vi "BRig_RT_panel_Laser2_v1,11.vi"(7 "input_setValues":bool, 9 "input_dataExp":u16[](array[numeric]), 11 "input_dataLC":u16[](array[numeric])) -> (1 "output_dataExp":u16[](array[numeric]), 3 "output_dataLC":u16[](array[numeric]))   [LabVIEW 2014]
panel:
  in  "LC_Sel_nRew2":u16
  in  "LC_Sel_nRew1":u16
  in  "LC_Cue2_nRew2":u16
  in  "LC_Cue2_nRew1":u16
  in  "LC_Cue_nRew2":u16
  in  "LC_Cue_nRew1":u16
  in  "LC_ENL2_nRew2":u16
  in  "LC_ENL2_nRew1":u16
  in  "LC_ENL_nRew2":u16
  in  "LC_ENL_nRew1":u16
  in  "LC_Cue2_PostR_Count":u16
  in  "LC_Cue2_PostR_delayOpt":bool
  in  "LC_Cue2_PostR_Probability":u16
  in  "LC_Cue2_PostR_Block":u16(slide) max=2 step=1 scale=0.0..2.0
  in  "LC_Cue2_PostR_OnOff":bool
  in  "LC_Cue2_PostR_Tdelay":u16
  in  "LC_ENL2_PostR_delayOpt":bool
  in  "LC_ENL2_PostR_Count":u16
  in  "LC_ENL2_PostR_Probability":u16 max=100 step=1
  in  "LC_ENL2_PostR_Block":u16(slide) max=2 step=1 scale=0.0..2.0
  in  "LC_ENL2_PostR_OnOff":bool
  in  "LC_ENL2_PostR_Tdelay":u16
  in  "LC_Cue2_PreR_Count":u16
  in  "LC_Cue2_First_Count":u16
  in  "LC_Cue2_PreR_delayOpt":bool
  in  "LC_ENL2_PreR_delayOpt":bool
  in  "LC_ENL2_PreR_Count":u16
  in  "LC_ENL2_First_Count":u16
  in  "LC_Cue2_First_delayOpt":bool
  in  "LC_ENL2_First_delayOpt":bool
  in  "LC_Cue2_PreR_Probability":u16
  in  "LC_Cue2_PreR_Block":u16(slide) max=2 step=1 scale=0.0..2.0
  in  "LC_Cue2_PreR_OnOff":bool
  in  "LC_Cue2_First_Probability":u16
  in  "LC_Cue2_First_Block":u16(slide) max=2 step=1 scale=0.0..2.0
  in  "LC_Cue2_First_OnOff":bool
  in  "LC_ENL2_PreR_Probability":u16 max=100 step=1
  in  "LC_ENL2_PreR_Block":u16(slide) max=2 step=1 scale=0.0..2.0
  in  "LC_ENL2_PreR_OnOff":bool
  in  "LC_ENL2_First_Probability":u16 max=100 step=1
  in  "LC_ENL2_First_Block":u16(slide) max=2 step=1 scale=0.0..2.0
  in  "LC_Cue2_PreR_Tdelay":u16
  in  "LC_ENL2_PreR_Tdelay":u16
  in  "LC_Cue2_First_Tdelay":u16
  in  "LC_ENL2_First_Tdelay":u16
  in  "LC_ENL2_First_OnOff":bool
  out "LaserPulseTrain":cluster{u16[], u16[]}(graph)
  in  "LED_baseline":bool
  in  "Laser_power_step":dbl
  in  "Laser_power_max":dbl
  in  "Laser_power_min":dbl
  in  "Laser_Tshutter":u16=2
  in  "Laser_Freq":u16=10
  in  "Laser_Tpeak":u16=2
  in  "Laser_T":u16
  in  "LC_Sel_PostR_Count":u16
  in  "LC_Sel_PostR_Probability":u16
  in  "LC_Sel_PostR_Block":u16(slide) max=2 step=1 scale=0.0..2.0
  in  "LC_Sel_PostR_OnOff":bool
  in  "LC_Sel_PostR_Tdelay":u16
  in  "LC_Cue_PostR_Count":u16
  in  "LC_Cue_PostR_delayOpt":bool
  in  "LC_Cue_PostR_Probability":u16
  in  "LC_Cue_PostR_Block":u16(slide) max=2 step=1 scale=0.0..2.0
  in  "LC_Cue_PostR_OnOff":bool
  in  "LC_Cue_PostR_Tdelay":u16
  in  "LC_ENL_PostR_delayOpt":bool
  in  "LC_ENL_PostR_Count":u16
  in  "LC_ENL_PostR_Probability":u16 max=100 step=1
  in  "LC_ENL_PostR_Block":u16(slide) max=2 step=1 scale=0.0..2.0
  in  "LC_ENL_PostR_OnOff":bool
  in  "LC_ENL_PostR_Tdelay":u16
  in  "LC_Sel_PreR_Count":u16
  in  "LC_Sel_First_Count":u16
  in  "LC_Sel_PreR_Probability":u16
  in  "LC_Sel_PreR_Block":u16(slide) max=2 step=1 scale=0.0..2.0
  in  "LC_Sel_PreR_OnOff":bool
  in  "LC_Sel_First_Probability":u16
  in  "LC_Sel_First_Block":u16(slide) max=2 step=1 scale=0.0..2.0
  in  "LC_Sel_First_OnOff":bool
  in  "LC_Sel_PreR_Tdelay":u16
  in  "LC_Sel_First_Tdelay":u16
  in  "LC_Cue_PreR_Count":u16
  in  "LC_Cue_First_Count":u16
  in  "LC_Cue_PreR_delayOpt":bool
  in  "LC_ENL_PreR_delayOpt":bool
  in  "LC_ENL_PreR_Count":u16
  in  "LC_ENL_First_Count":u16
  in  "LC_Cue_First_delayOpt":bool
  in  "LC_ENL_First_delayOpt":bool
  in  "LC_Wrong_Probability":u16
  in  "LC_Wrong_Trial":u16(slide) max=2 step=1 scale=0.0..2.0
  in  "LC_Wrong_Block":u16(slide) max=2 step=1 scale=0.0..2.0
  in  "LC_Wrong_OnOff":bool
  in  "LC_Reward_Probability":u16
  in  "LC_Reward_Trial":u16(slide) max=2 step=1 scale=0.0..2.0
  in  "LC_Reward_Block":u16(slide) max=2 step=1 scale=0.0..2.0
  in  "LC_Reward_OnOff":bool
  in  "LC_Cue_PreR_Probability":u16
  in  "LC_Cue_PreR_Block":u16(slide) max=2 step=1 scale=0.0..2.0
  in  "LC_Cue_PreR_OnOff":bool
  in  "LC_Cue_First_Probability":u16
  in  "LC_Cue_First_Block":u16(slide) max=2 step=1 scale=0.0..2.0
  in  "LC_Cue_First_OnOff":bool
  in  "LC_ENL_PreR_Probability":u16 max=100 step=1
  in  "LC_ENL_PreR_Block":u16(slide) max=2 step=1 scale=0.0..2.0
  in  "LC_ENL_PreR_OnOff":bool
  in  "LC_ENL_First_Probability":u16 max=100 step=1
  in  "LC_ENL_First_Block":u16(slide) max=2 step=1 scale=0.0..2.0
  in  "LC_Wrong_Tdelay":u16
  in  "LC_Cue_PreR_Tdelay":u16
  in  "LC_ENL_PreR_Tdelay":u16
  in  "LC_Reward_Tdelay":u16
  in  "LC_Cue_First_Tdelay":u16
  in  "LC_ENL_First_Tdelay":u16
  in  "LC_ENL_First_OnOff":bool
  # "Laser2 Control\n                               On/Off      Block        Probability [%]   Delay [ms]                              Count"
  # "On/Off      Block        Probability [%]   Delay [ms]                              Count"
  # "Enforced\nNonLick"
  # "Enforced\nNonLick\n     2"
  # "from end"
  # "from end"
  # "First\nTrial"
  # "First\nTrial"
  # "from start"
  # "from start"
  # "from end"
  # "from end"
  # "PreReward\nTrials"
  # "PreReward\nTrials"
  # "from start"
  # "from start"
  # "from end"
  # "from end"
  # "PostReward\nTrials"
  # "PostReward\nTrials"
  # "from start"
  # "from start"
  # "PostReward Option - Trigger after [X1] or [X2] reward\n                                        (0 = ignore this option)"
  # "PostReward Option - Trigger after [X1] or [X2] reward\n                                        (0 = ignore this option)"
  # "Cue"
  # "Cue\n  2"
  # "from end"
  # "from end"
  # "First\nTrial"
  # "First\nTrial"
  # "from start"
  # "from start"
  # "from end"
  # "from end"
  # "PreReward\nTrials"
  # "PreReward\nTrials"
  # "from start"
  # "from start"
  # "from end"
  # "from end"
  # "PostReward\nTrials"
  # "PostReward\nTrials"
  # "from start"
  # "from start"
  # "PostReward Option - Trigger after [X1] or [X2] reward\n                                        (0 = ignore this option)"
  # "PostReward Option - Trigger after [X1] or [X2] reward\n                                        (0 = ignore this option)"
  # "Selection"
  # "from start"
  # "First\nTrial"
  # "from start"
  # "PreReward\nTrials"
  # "from start"
  # "PostReward\nTrials"
  # "PostReward Option - Trigger after [X1] or [X2] reward\n                                        (0 = ignore this option)"
  # "Laser2 Parameters"
  # "Laser2 Response\n           On/Off      Block           Trial     Probability %  Delay [ms]"
  # "Frequency\n[Hz]"
  # "Selection\nReward"
  # "Timing [ms]\n Duration     Peak Width   Shutter"
  # "Selection\nWrong"
  # "Laser Power [V]\nMin          Max              Step"
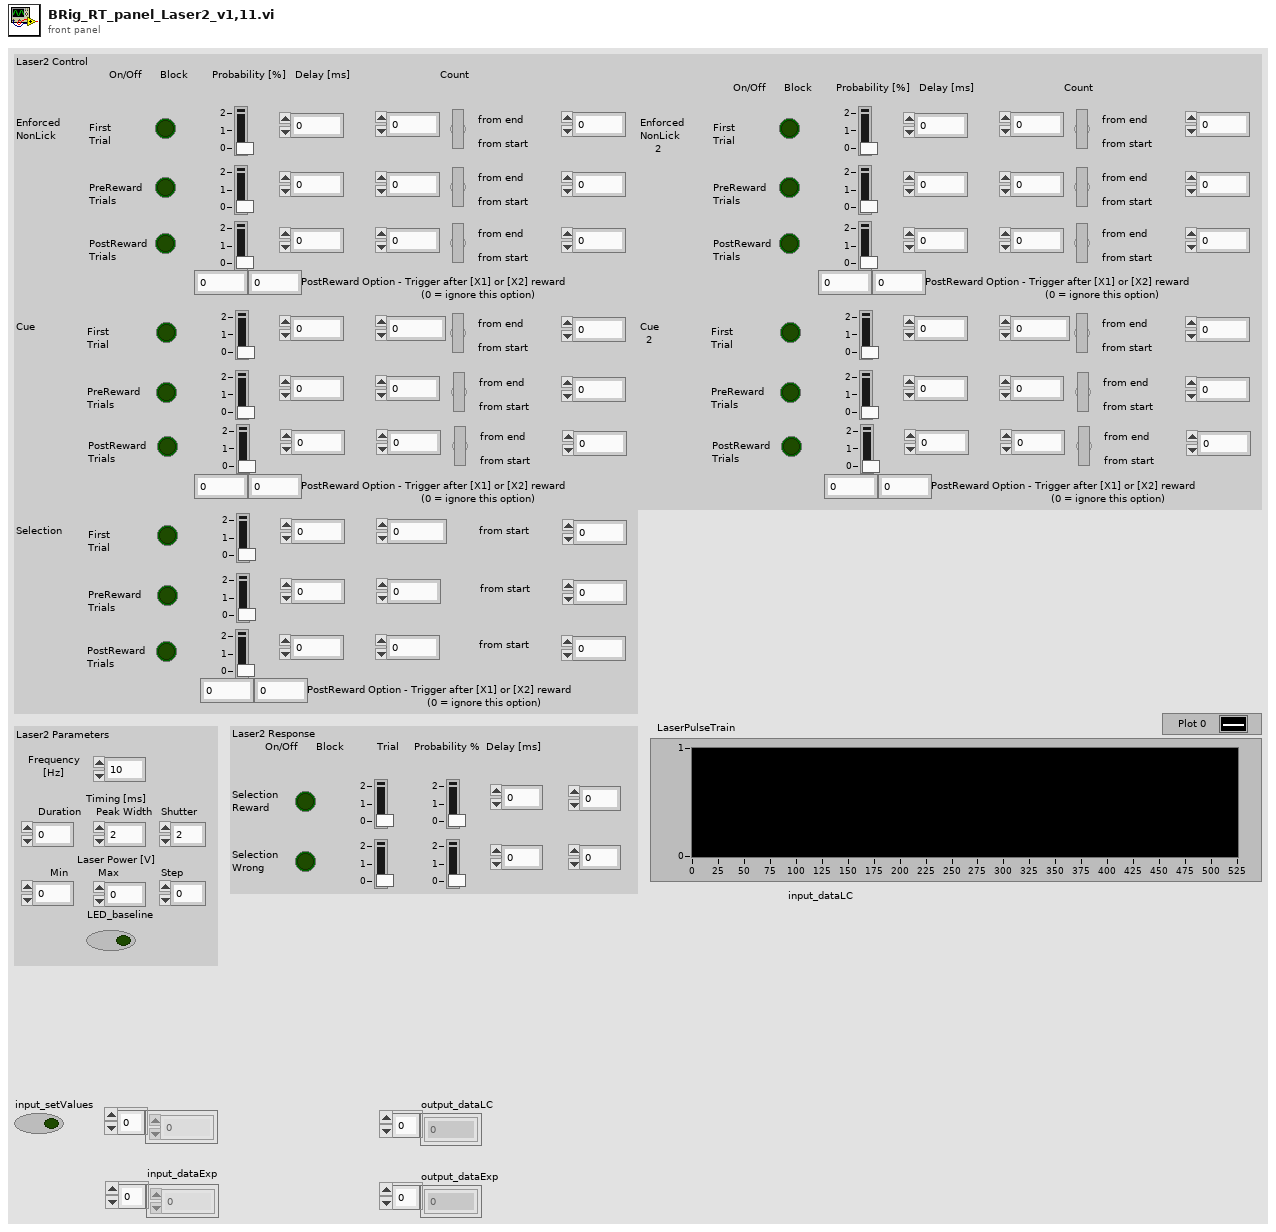
[diagram p1: front panel]
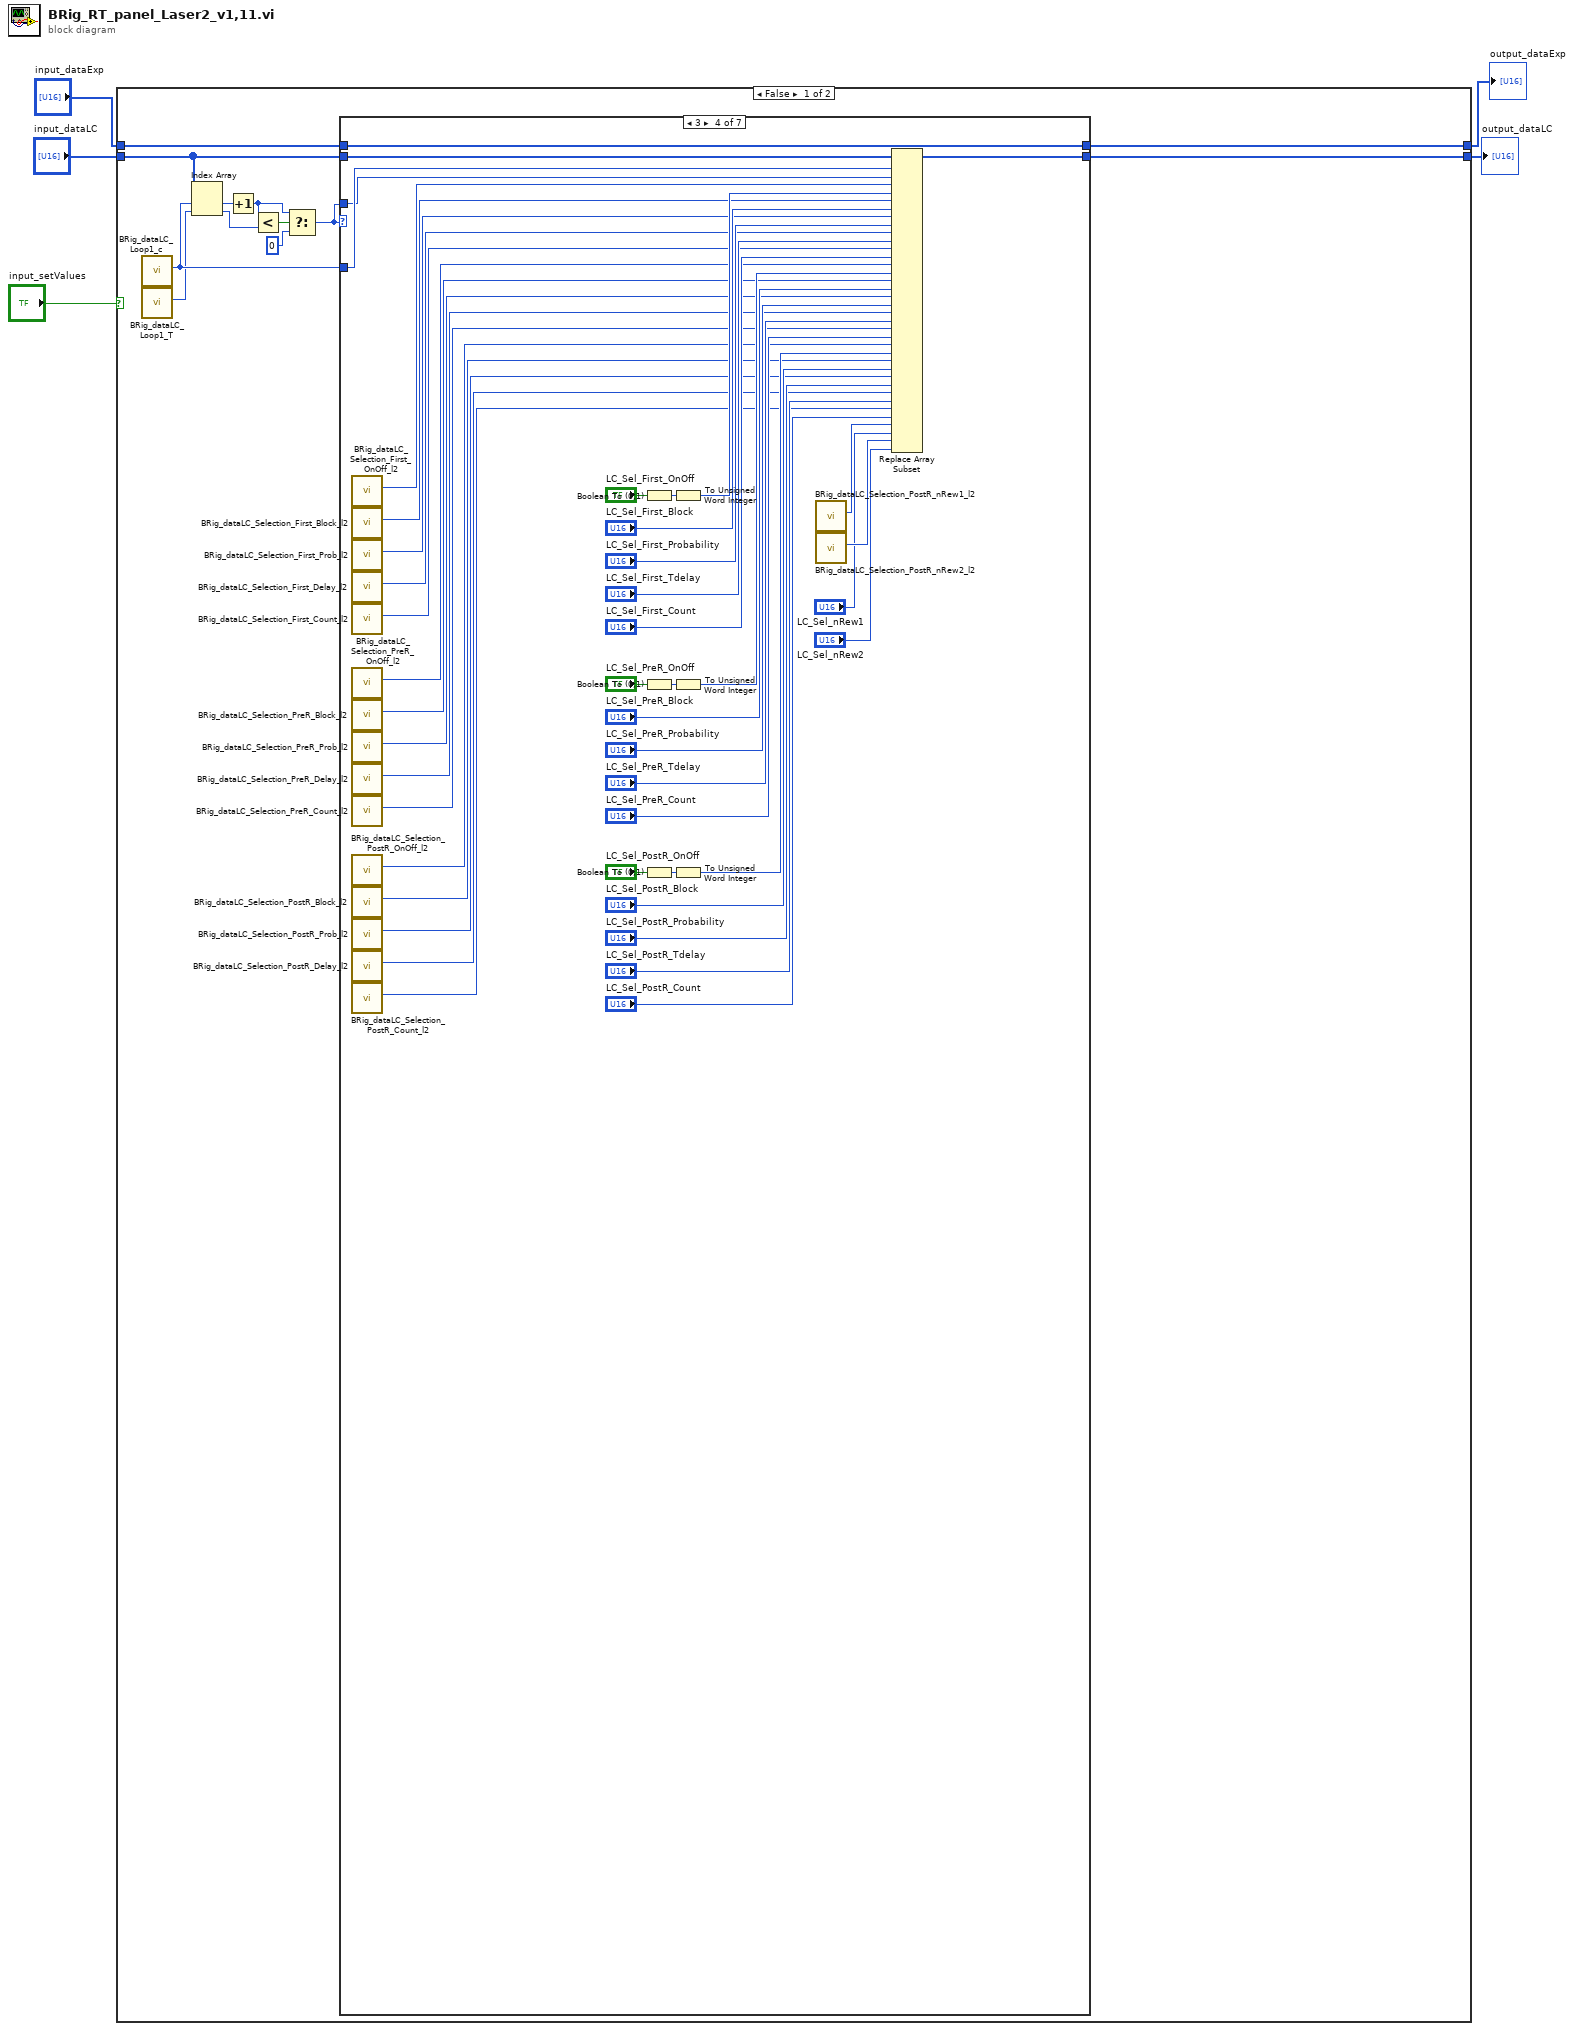
[diagram p0: block diagram]
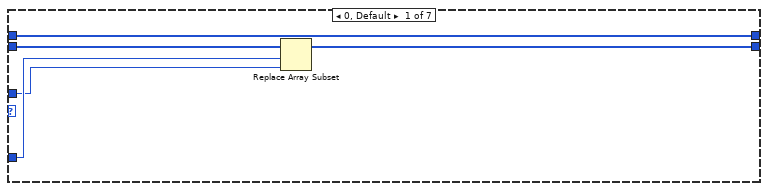
[diagram p2: hidden frame]
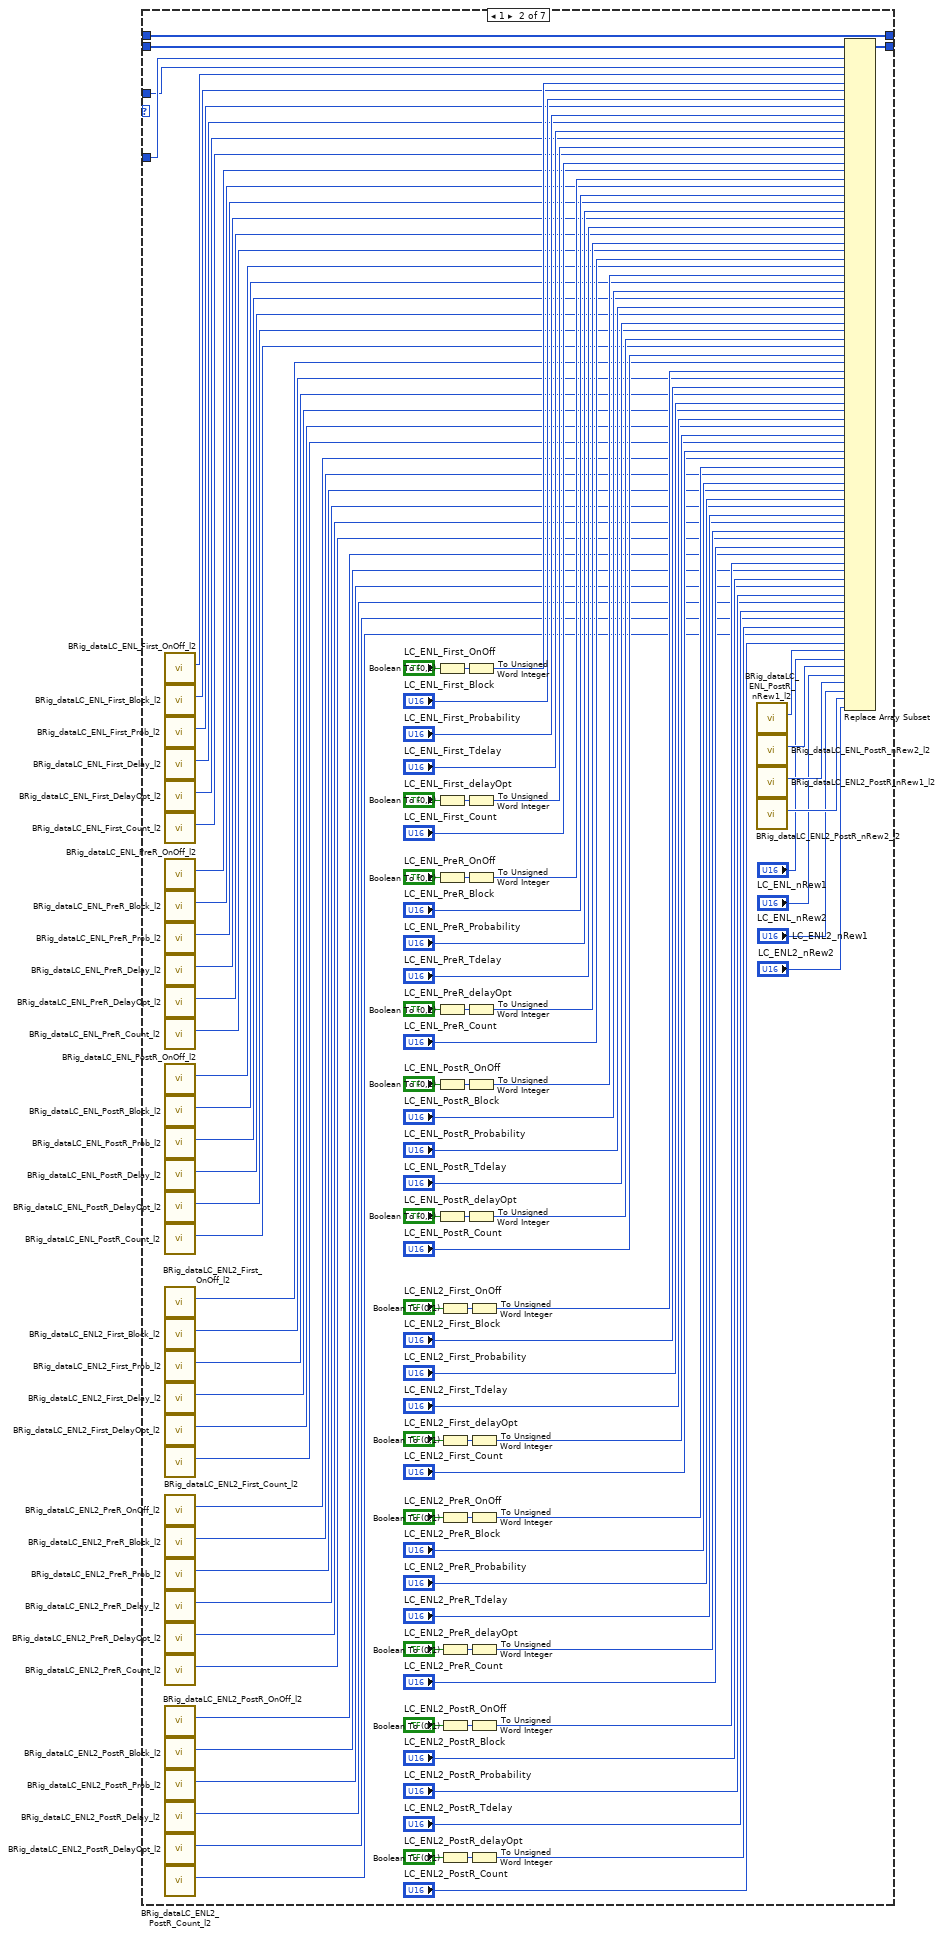
[diagram p3: hidden frame]
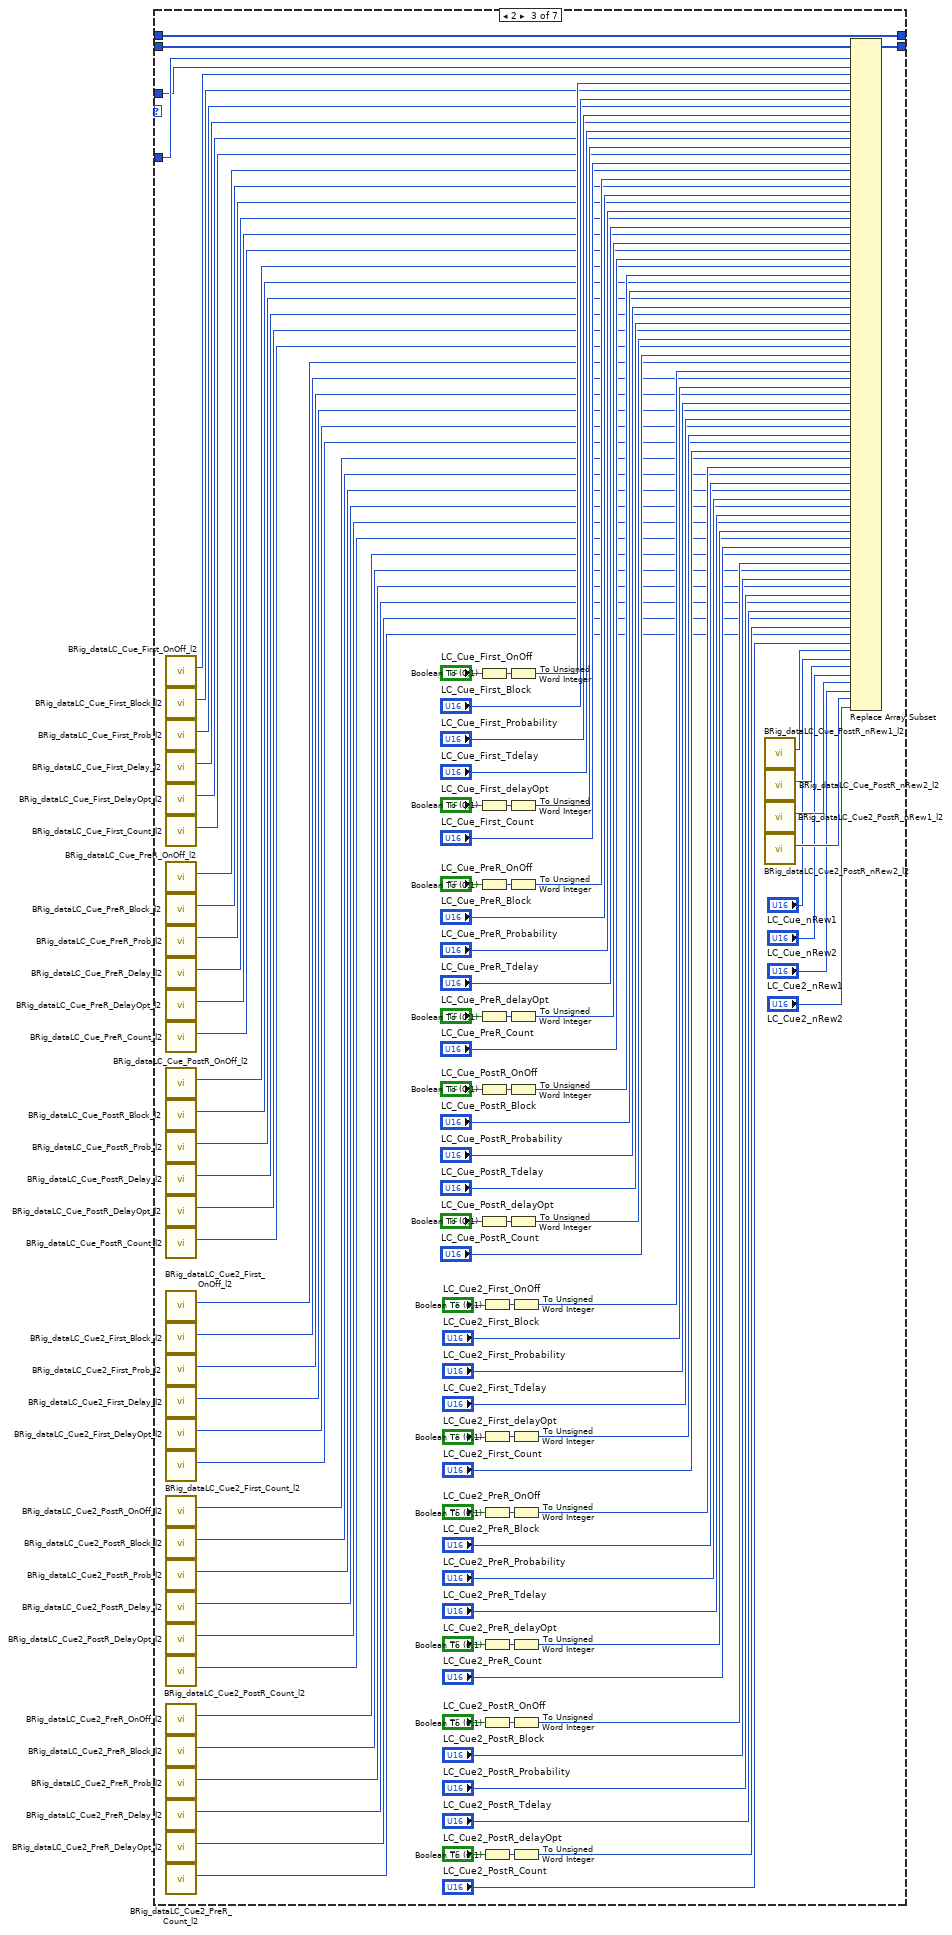
[diagram p4: hidden frame]
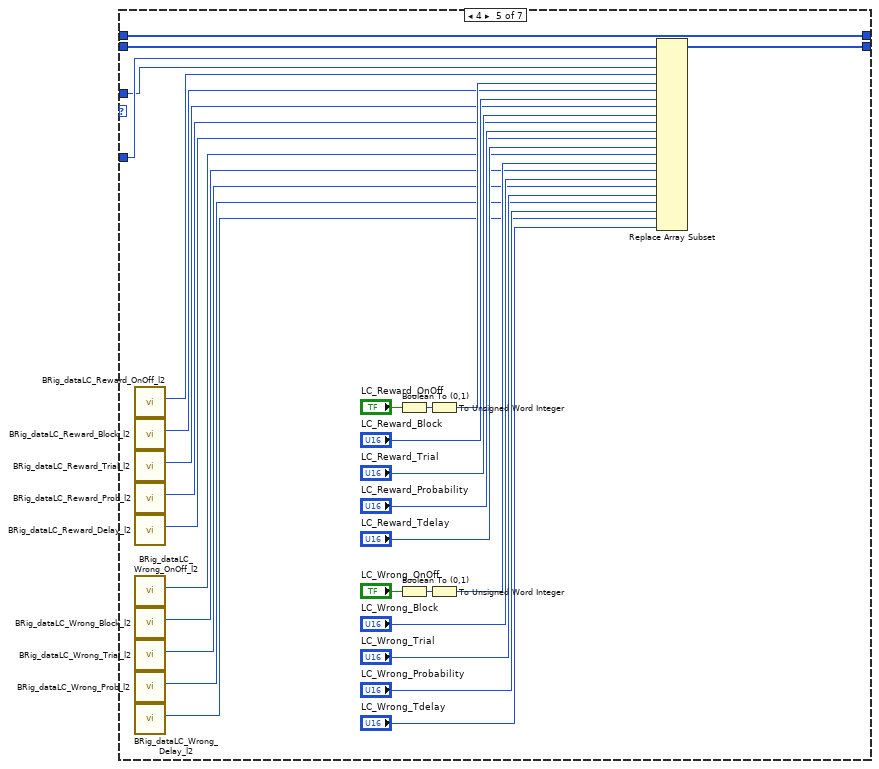
[diagram p5: hidden frame]
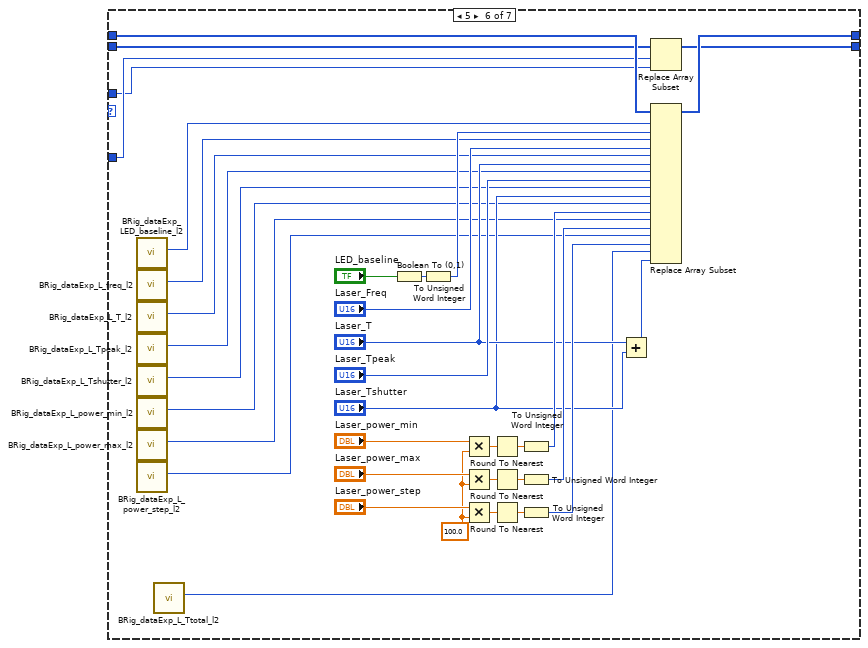
[diagram p6: hidden frame]
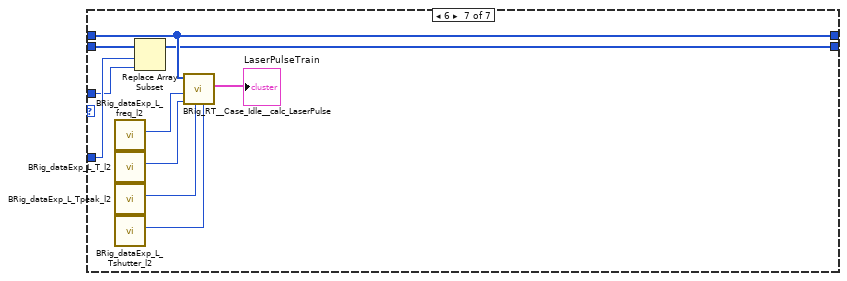
[diagram p7: hidden frame]
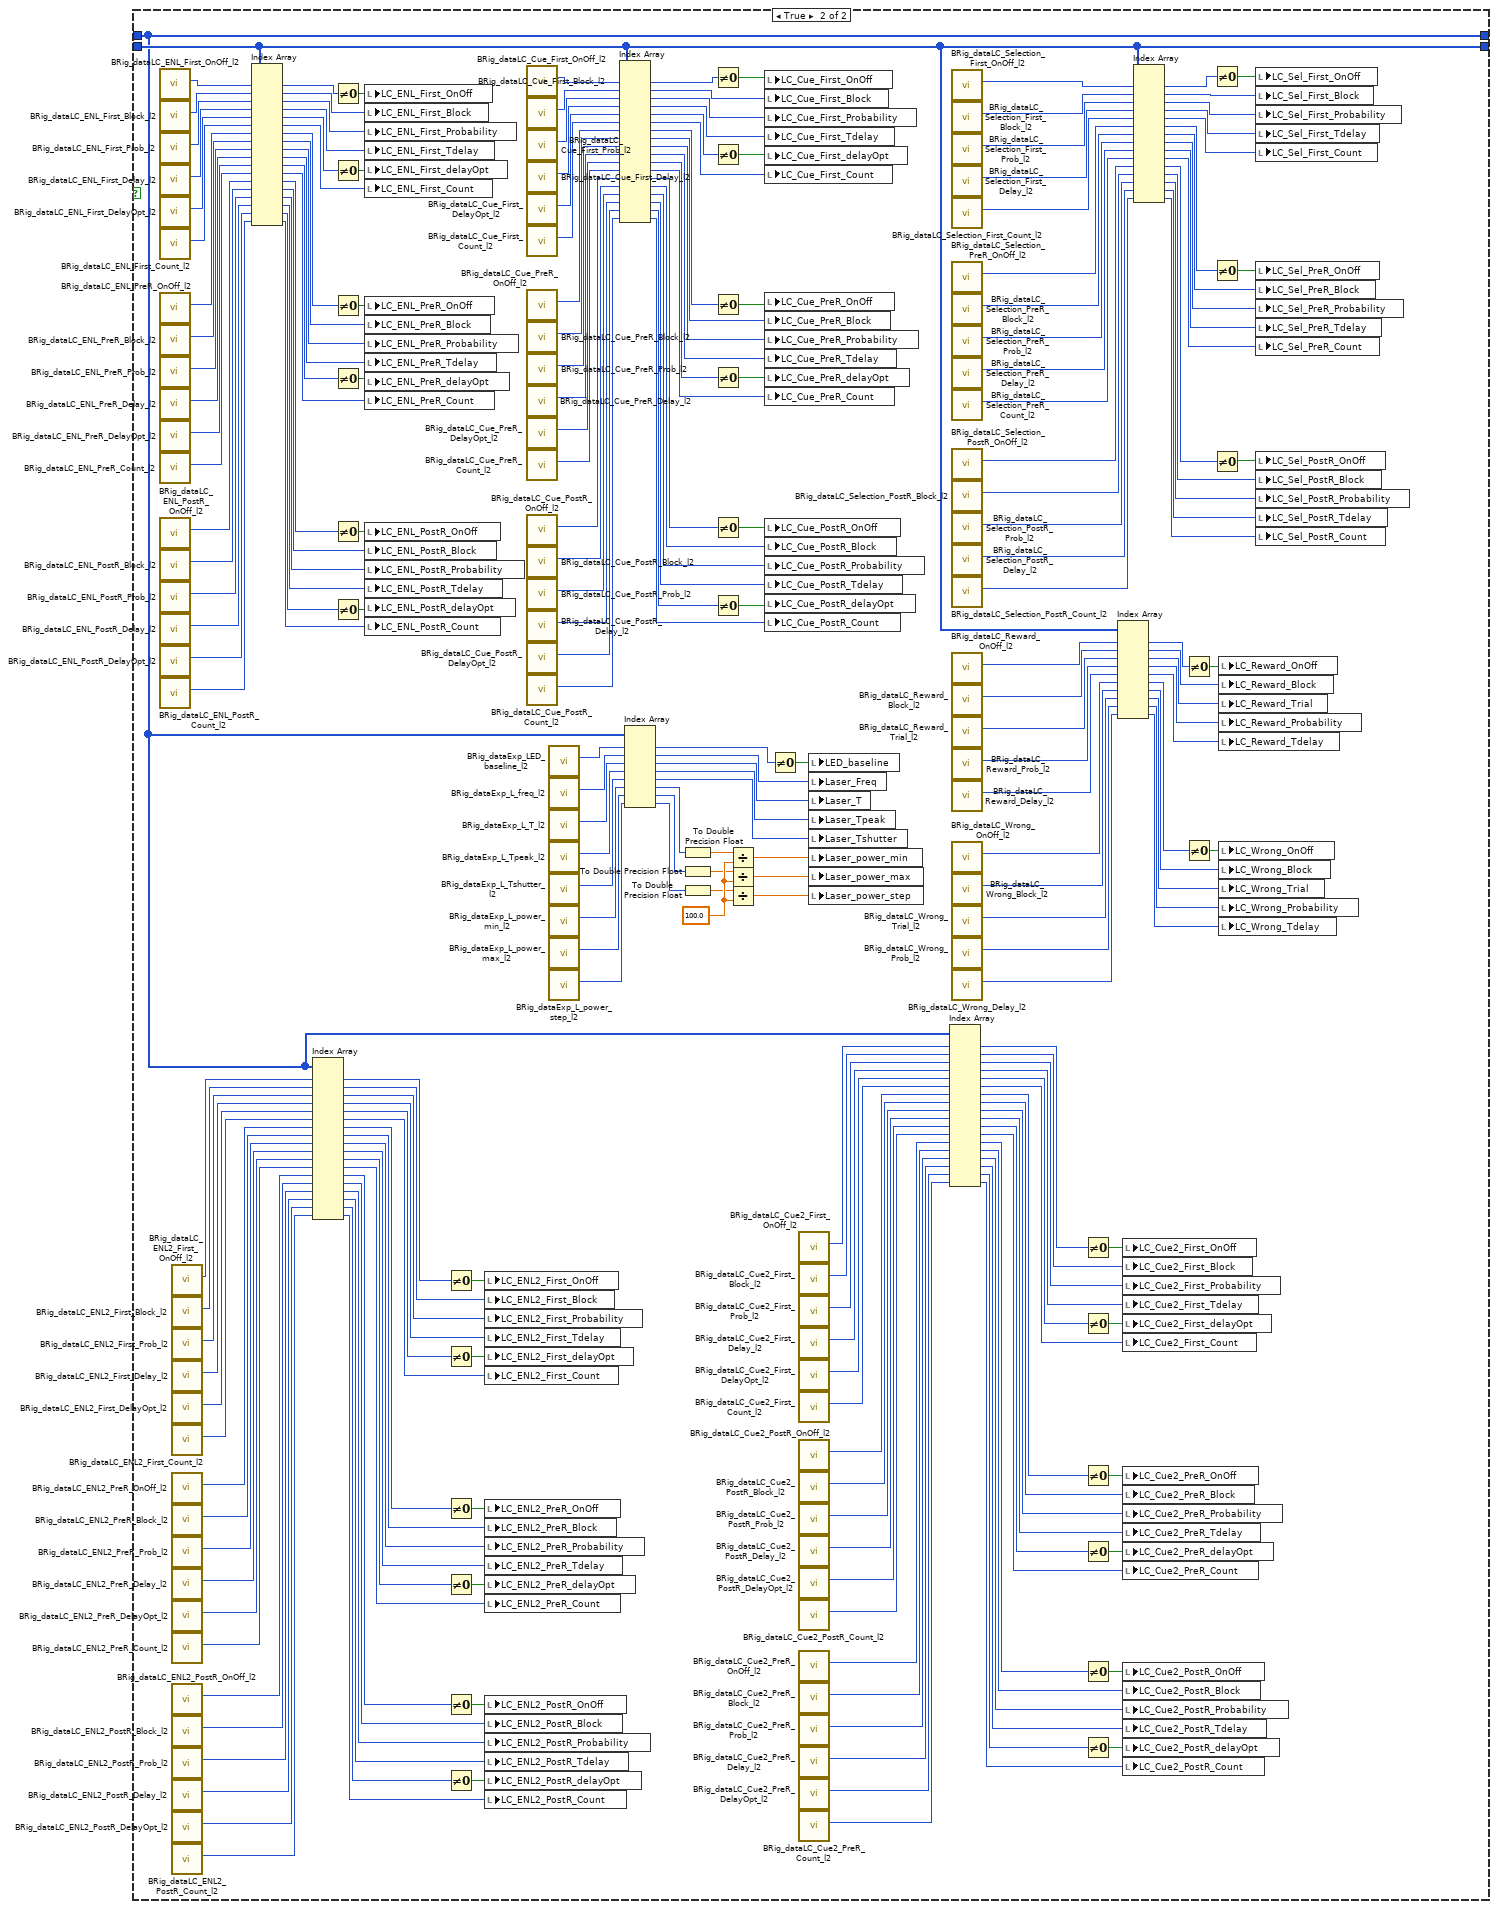
[diagram p8: hidden frame]
diagram:
  n1 = case shown="False" "input_setValues" {
    tunnel: "input_dataLC" -> [w17 w531]
    tunnel: [w11 w531] -> w4
    tunnel: "input_dataExp" -> [w7 w484]
    tunnel: [w6 w484] -> w1
    frame False {
      n2 = call "BRig_dataLC_Loop1_c.vi"() -> ("output_Loop1_c"=w10:i32)  [unwired: 11 in]
      n3 = call "BRig_dataLC_Loop1_T.vi"() -> ("output_Loop1_T"=w9:i32)  [unwired: 11 in]
      n4 = Index Array(array=w17, index #1=w10, index #2=w9) -> (element #1=w16:u16, element #2=w15:u16)
      n5 = Increment(x=w16) -> (x+1=w12:u16)
      n6 = Less?(x=w12, y=w15) -> (x < y?=w14:bool)
      n7 = Select(t=w12, s=w14, f=u16 0) -> (s? t:f=w8:u16)
      n8 = case shown="3" w8 {
        tunnel: w17 -> [w22 w131 w240 w285 w314 w327 w358]
        tunnel: w10 -> [w20 w99 w208 w262 w298 w325 w356]
        tunnel: w8 -> [w19 w98 w207 w261 w297 w324 w355]
        tunnel: [w21 w130 w239 w284 w313 w326 w357] -> w11
        tunnel: w7 -> [w18 w97 w206 w260 w296 w329 w360]
        tunnel: [w18 w97 w206 w260 w296 w328 w360] -> w6
        frame 0, Default {
          n9 = Replace Array Subset(array=w22, new element=w19, index=w20) -> (w21:u16[])
        }
        frame 1 {
          n10 = call "BRig_dataLC_ENL_First_OnOff_l2.vi"() -> ("output_ENL_First_OnOff_l2"=w49:i32)  [unwired: 11 in]
          n11 = call "BRig_dataLC_ENL_First_Block_l2.vi"() -> ("output_ENL_First_Block_l2"=w50:i32)  [unwired: 11 in]
          n12 = call "BRig_dataLC_ENL_First_Prob_l2.vi"() -> ("output_ENL_First_Prob_l2"=w51:i32)  [unwired: 11 in]
          n13 = call "BRig_dataLC_ENL_First_Delay_l2.vi"() -> ("output_ENL_First_Delay_l2"=w52:i32)  [unwired: 11 in]
          n14 = call "BRig_dataLC_ENL_First_DelayOpt_l2.vi"() -> ("output_ENL_First_DelayOpt_l2"=w53:i32)  [unwired: 11 in]
          n15 = call "BRig_dataLC_ENL_First_Count_l2.vi"() -> ("output_ENL_First_Count_l2"=w54:i32)  [unwired: 11 in]
          n16 = call "BRig_dataLC_ENL_PreR_OnOff_l2.vi"() -> ("output_ENL_PreR_OnOff_l2"=w55:i32)  [unwired: 11 in]
          n17 = call "BRig_dataLC_ENL_PreR_Block_l2.vi"() -> ("output_ENL_PreR_Block_l2"=w56:i32)  [unwired: 11 in]
          n18 = call "BRig_dataLC_ENL_PreR_Prob_l2.vi"() -> ("output_ENL_PreR_Prob_l2"=w57:i32)  [unwired: 11 in]
          n19 = call "BRig_dataLC_ENL_PreR_Delay_l2.vi"() -> ("output_ENL_PreR_Delay_l2"=w58:i32)  [unwired: 11 in]
          n20 = call "BRig_dataLC_ENL_PreR_DelayOpt_l2.vi"() -> ("output_ENL_PreR_DelayOpt_l2"=w59:i32)  [unwired: 11 in]
          n21 = call "BRig_dataLC_ENL_PreR_Count_l2.vi"() -> ("output_ENL_PreR_Count_l2"=w60:i32)  [unwired: 11 in]
          n22 = call "BRig_dataLC_ENL_PostR_OnOff_l2.vi"() -> ("output_ENL_PostR_OnOff_l2"=w61:i32)  [unwired: 11 in]
          n23 = call "BRig_dataLC_ENL_PostR_Block_l2.vi"() -> ("output_ENL_PostR_Block_l2"=w62:i32)  [unwired: 11 in]
          n24 = call "BRig_dataLC_ENL_PostR_Prob_l2.vi"() -> ("output_ENL_PostR_Prob_l2"=w63:i32)  [unwired: 11 in]
          n25 = call "BRig_dataLC_ENL_PostR_Delay_l2.vi"() -> ("output_ENL_PostR_Delay_l2"=w64:i32)  [unwired: 11 in]
          n26 = call "BRig_dataLC_ENL_PostR_DelayOpt_l2.vi"() -> ("output_ENL_PostR_DelayOpt_l2"=w65:i32)  [unwired: 11 in]
          n27 = call "BRig_dataLC_ENL_PostR_Count_l2.vi"() -> ("output_ENL_PostR_Count_l2"=w66:i32)  [unwired: 11 in]
          n28 = call "BRig_dataLC_ENL2_First_OnOff_l2.vi"() -> ("output_ENL2_First_OnOff_l2"=w48:i32)  [unwired: 11 in]
          n29 = call "BRig_dataLC_ENL2_First_Block_l2.vi"() -> ("output_ENL2_First_Block_l2"=w47:i32)  [unwired: 11 in]
          n30 = call "BRig_dataLC_ENL2_First_Prob_l2.vi"() -> ("output_ENL2_First_Prob_l2"=w46:i32)  [unwired: 11 in]
          n31 = call "BRig_dataLC_ENL2_First_Delay_l2.vi"() -> ("output_ENL2_First_Delay_l2"=w45:i32)  [unwired: 11 in]
          n32 = call "BRig_dataLC_ENL2_First_DelayOpt_l2.vi"() -> ("output_ENL2_First_DelayOpt_l2"=w44:i32)  [unwired: 11 in]
          n33 = call "BRig_dataLC_ENL2_First_Count_l2.vi"() -> ("output_ENL2_First_Count_l2"=w43:i32)  [unwired: 11 in]
          n34 = call "BRig_dataLC_ENL2_PreR_OnOff_l2.vi"() -> ("output_ENL2_PreR_OnOff_l2"=w42:i32)  [unwired: 11 in]
          n35 = call "BRig_dataLC_ENL2_PreR_Block_l2.vi"() -> ("output_ENL2_PreR_Block_l2"=w41:i32)  [unwired: 11 in]
          n36 = call "BRig_dataLC_ENL2_PreR_Prob_l2.vi"() -> ("output_ENL2_PreR_Prob_l2"=w40:i32)  [unwired: 11 in]
          n37 = call "BRig_dataLC_ENL2_PreR_Delay_l2.vi"() -> ("output_ENL2_PreR_Delay_l2"=w39:i32)  [unwired: 11 in]
          n38 = call "BRig_dataLC_ENL2_PreR_DelayOpt_l2.vi"() -> ("output_ENL2_PreR_DelayOpt_l2"=w38:i32)  [unwired: 11 in]
          n39 = call "BRig_dataLC_ENL2_PreR_Count_l2.vi"() -> ("output_ENL2_PreR_Count_l2"=w37:i32)  [unwired: 11 in]
          n40 = call "BRig_dataLC_ENL2_PostR_OnOff_l2.vi"() -> ("output_ENL2_PostR_OnOff_l2"=w36:i32)  [unwired: 11 in]
          n41 = call "BRig_dataLC_ENL2_PostR_Block_l2.vi"() -> ("output_ENL2_PostR_Block_l2"=w35:i32)  [unwired: 11 in]
          n42 = call "BRig_dataLC_ENL2_PostR_Prob_l2.vi"() -> ("output_ENL2_PostR_Prob_l2"=w34:i32)  [unwired: 11 in]
          n43 = call "BRig_dataLC_ENL2_PostR_Delay_l2.vi"() -> ("output_ENL2_PostR_Delay_l2"=w33:i32)  [unwired: 11 in]
          n44 = call "BRig_dataLC_ENL2_PostR_DelayOpt_l2.vi"() -> ("output_ENL2_PostR_DelayOpt_l2"=w32:i32)  [unwired: 11 in]
          n45 = call "BRig_dataLC_ENL2_PostR_Count_l2.vi"() -> ("output_ENL2_PostR_Count_l2"=w31:i32)  [unwired: 11 in]
          n46 = Boolean To (0,1)(Boolean="LC_ENL_First_OnOff") -> (0, 1=w128:i16)
          n47 = Boolean To (0,1)(Boolean="LC_ENL_First_delayOpt") -> (0, 1=w127:i16)
          n48 = Boolean To (0,1)(Boolean="LC_ENL_PreR_OnOff") -> (0, 1=w125:i16)
          n49 = Boolean To (0,1)(Boolean="LC_ENL_PreR_delayOpt") -> (0, 1=w123:i16)
          n50 = Boolean To (0,1)(Boolean="LC_ENL_PostR_OnOff") -> (0, 1=w121:i16)
          n51 = Boolean To (0,1)(Boolean="LC_ENL_PostR_delayOpt") -> (0, 1=w119:i16)
          n52 = Boolean To (0,1)(Boolean="LC_ENL2_First_OnOff") -> (0, 1=w87:i16)
          n53 = Boolean To (0,1)(Boolean="LC_ENL2_First_delayOpt") -> (0, 1=w86:i16)
          n54 = Boolean To (0,1)(Boolean="LC_ENL2_PreR_OnOff") -> (0, 1=w85:i16)
          n55 = Boolean To (0,1)(Boolean="LC_ENL2_PreR_delayOpt") -> (0, 1=w83:i16)
          n56 = Boolean To (0,1)(Boolean="LC_ENL2_PostR_OnOff") -> (0, 1=w75:i16)
          n57 = Boolean To (0,1)(Boolean="LC_ENL2_PostR_delayOpt") -> (0, 1=w73:i16)
          n58 = To Unsigned Word Integer(number=w128) -> (unsigned 16bit integer=w117:u16)
          n59 = To Unsigned Word Integer(number=w127) -> (unsigned 16bit integer=w113:u16)
          n60 = To Unsigned Word Integer(number=w125) -> (unsigned 16bit integer=w111:u16)
          n61 = To Unsigned Word Integer(number=w123) -> (unsigned 16bit integer=w107:u16)
          n62 = To Unsigned Word Integer(number=w121) -> (unsigned 16bit integer=w105:u16)
          n63 = To Unsigned Word Integer(number=w119) -> (unsigned 16bit integer=w101:u16)
          n64 = To Unsigned Word Integer(number=w87) -> (unsigned 16bit integer=w94:u16)
          n65 = To Unsigned Word Integer(number=w86) -> (unsigned 16bit integer=w90:u16)
          n66 = To Unsigned Word Integer(number=w85) -> (unsigned 16bit integer=w88:u16)
          n67 = To Unsigned Word Integer(number=w83) -> (unsigned 16bit integer=w78:u16)
          n68 = To Unsigned Word Integer(number=w75) -> (unsigned 16bit integer=w76:u16)
          n69 = To Unsigned Word Integer(number=w73) -> (unsigned 16bit integer=w68:u16)
          n70 = call "BRig_dataLC_ENL_PostR_nRew1_l2.vi"() -> ("output_ENL_PostR_nRew1_l2"=w30:i32)  [unwired: 11 in]
          n71 = call "BRig_dataLC_ENL_PostR_nRew2_l2.vi"() -> ("output_ENL_PostR_nRew2_l2"=w29:i32)  [unwired: 11 in]
          n72 = call "BRig_dataLC_ENL2_PostR_nRew1_l2.vi"() -> ("output_ENL2_PostR_nRew1_l2"=w28:i32)  [unwired: 11 in]
          n73 = call "BRig_dataLC_ENL2_PostR_nRew2_l2.vi"() -> ("output_ENL2_PostR_nRew2_l2"=w27:i32)  [unwired: 11 in]
          n74 = Replace Array Subset(array=w131, new element #1=w98, index #1=w99, new element #2=w117, index #2=w49, new element #3="LC_ENL_First_Block", index #3=w50, new element #4="LC_ENL_First_Probability", index #4=w51, new element #5="LC_ENL_First_Tdelay", index #5=w52, new element #6=w113, index #6=w53, new element #7="LC_ENL_First_Count", index #7=w54, new element #8=w111, index #8=w55, new element #9="LC_ENL_PreR_Block", index #9=w56, new element #10="LC_ENL_PreR_Probability", index #10=w57, new element #11="LC_ENL_PreR_Tdelay", index #11=w58, new element #12=w107, index #12=w59, new element #13="LC_ENL_PreR_Count", index #13=w60, new element #14=w105, index #14=w61, new element #15="LC_ENL_PostR_Block", index #15=w62, new element #16="LC_ENL_PostR_Probability", index #16=w63, new element #17="LC_ENL_PostR_Tdelay", index #17=w64, new element #18=w101, index #18=w65, new element #19="LC_ENL_PostR_Count", index #19=w66, new element #20=w94, index #20=w48, new element #21="LC_ENL2_First_Block", index #21=w47, new element #22="LC_ENL2_First_Probability", index #22=w46, new element #23="LC_ENL2_First_Tdelay", index #23=w45, new element #24=w90, index #24=w44, new element #25="LC_ENL2_First_Count", index #25=w43, new element #26=w88, index #26=w42, new element #27="LC_ENL2_PreR_Block", index #27=w41, new element #28="LC_ENL2_PreR_Probability", index #28=w40, new element #29="LC_ENL2_PreR_Tdelay", index #29=w39, new element #30=w78, index #30=w38, new element #31="LC_ENL2_PreR_Count", index #31=w37, new element #32=w76, index #32=w36, new element #33="LC_ENL2_PostR_Block", index #33=w35, new element #34="LC_ENL2_PostR_Probability", index #34=w34, new element #35="LC_ENL2_PostR_Tdelay", index #35=w33, new element #36=w68, index #36=w32, new element #37="LC_ENL2_PostR_Count", index #37=w31, new element #38="LC_ENL_nRew1", index #38=w30, new element #39="LC_ENL_nRew2", index #39=w29, new element #40="LC_ENL2_nRew1", index #40=w28, new element #41="LC_ENL2_nRew2", index #41=w27) -> (w130:u16[])
        }
        frame 2 {
          n75 = call "BRig_dataLC_Cue_First_OnOff_l2.vi"() -> ("output_Cue_First_OnOff_l2"=w158:i32)  [unwired: 11 in]
          n76 = call "BRig_dataLC_Cue_First_Block_l2.vi"() -> ("output_Cue_First_Block_l2"=w159:i32)  [unwired: 11 in]
          n77 = call "BRig_dataLC_Cue_First_Prob_l2.vi"() -> ("output_Cue_First_Prob_l2"=w160:i32)  [unwired: 11 in]
          n78 = call "BRig_dataLC_Cue_First_Delay_l2.vi"() -> ("output_Cue_First_Delay_l2"=w161:i32)  [unwired: 11 in]
          n79 = call "BRig_dataLC_Cue_First_DelayOpt_l2.vi"() -> ("output_Cue_First_DelayOpt_l2"=w162:i32)  [unwired: 11 in]
          n80 = call "BRig_dataLC_Cue_First_Count_l2.vi"() -> ("output_Cue_First_Count_l2"=w163:i32)  [unwired: 11 in]
          n81 = call "BRig_dataLC_Cue_PreR_OnOff_l2.vi"() -> ("output_Cue_PreR_OnOff_l2"=w164:i32)  [unwired: 11 in]
          n82 = call "BRig_dataLC_Cue_PreR_Block_l2.vi"() -> ("output_Cue_PreR_Block_l2"=w165:i32)  [unwired: 11 in]
          n83 = call "BRig_dataLC_Cue_PreR_Prob_l2.vi"() -> ("output_Cue_PreR_Prob_l2"=w166:i32)  [unwired: 11 in]
          n84 = call "BRig_dataLC_Cue_PreR_Delay_l2.vi"() -> ("output_Cue_PreR_Delay_l2"=w167:i32)  [unwired: 11 in]
          n85 = call "BRig_dataLC_Cue_PreR_DelayOpt_l2.vi"() -> ("output_Cue_PreR_DelayOpt_l2"=w168:i32)  [unwired: 11 in]
          n86 = call "BRig_dataLC_Cue_PreR_Count_l2.vi"() -> ("output_Cue_PreR_Count_l2"=w169:i32)  [unwired: 11 in]
          n87 = call "BRig_dataLC_Cue_PostR_OnOff_l2.vi"() -> ("output_Cue_PostR_OnOff_l2"=w170:i32)  [unwired: 11 in]
          n88 = call "BRig_dataLC_Cue_PostR_Block_l2.vi"() -> ("output_Cue_PostR_Block_l2"=w171:i32)  [unwired: 11 in]
          n89 = call "BRig_dataLC_Cue_PostR_Prob_l2.vi"() -> ("output_Cue_PostR_Prob_l2"=w172:i32)  [unwired: 11 in]
          n90 = call "BRig_dataLC_Cue_PostR_Delay_l2.vi"() -> ("output_Cue_PostR_Delay_l2"=w173:i32)  [unwired: 11 in]
          n91 = call "BRig_dataLC_Cue_PostR_DelayOpt_l2.vi"() -> ("output_Cue_PostR_DelayOpt_l2"=w174:i32)  [unwired: 11 in]
          n92 = call "BRig_dataLC_Cue_PostR_Count_l2.vi"() -> ("output_Cue_PostR_Count_l2"=w175:i32)  [unwired: 11 in]
          n93 = call "BRig_dataLC_Cue2_First_OnOff_l2.vi"() -> ("output_Cue2_First_OnOff_l2"=w157:i32)  [unwired: 11 in]
          n94 = call "BRig_dataLC_Cue2_First_Block_l2.vi"() -> ("output_Cue2_First_Block_l2"=w156:i32)  [unwired: 11 in]
          n95 = call "BRig_dataLC_Cue2_First_Prob_l2.vi"() -> ("output_Cue2_First_Prob_l2"=w155:i32)  [unwired: 11 in]
          n96 = call "BRig_dataLC_Cue2_First_Delay_l2.vi"() -> ("output_Cue2_First_Delay_l2"=w154:i32)  [unwired: 11 in]
          n97 = call "BRig_dataLC_Cue2_First_DelayOpt_l2.vi"() -> ("output_Cue2_First_DelayOpt_l2"=w153:i32)  [unwired: 11 in]
          n98 = call "BRig_dataLC_Cue2_First_Count_l2.vi"() -> ("output_Cue2_First_Count_l2"=w152:i32)  [unwired: 11 in]
          n99 = call "BRig_dataLC_Cue2_PostR_OnOff_l2.vi"() -> ("output_Cue2_PostR_OnOff_l2"=w151:i32)  [unwired: 11 in]
          n100 = call "BRig_dataLC_Cue2_PostR_Block_l2.vi"() -> ("output_Cue2_PostR_Block_l2"=w150:i32)  [unwired: 11 in]
          n101 = call "BRig_dataLC_Cue2_PostR_Prob_l2.vi"() -> ("output_Cue2_PostR_Prob_l2"=w149:i32)  [unwired: 11 in]
          n102 = call "BRig_dataLC_Cue2_PostR_Delay_l2.vi"() -> ("output_Cue2_PostR_Delay_l2"=w148:i32)  [unwired: 11 in]
          n103 = call "BRig_dataLC_Cue2_PostR_DelayOpt_l2.vi"() -> ("output_Cue2_PostR_DelayOpt_l2"=w147:i32)  [unwired: 11 in]
          n104 = call "BRig_dataLC_Cue2_PostR_Count_l2.vi"() -> ("output_Cue2_PostR_Count_l2"=w146:i32)  [unwired: 11 in]
          n105 = call "BRig_dataLC_Cue2_PreR_OnOff_l2.vi"() -> ("output_Cue2_PreR_OnOff_l2"=w145:i32)  [unwired: 11 in]
          n106 = call "BRig_dataLC_Cue2_PreR_Block_l2.vi"() -> ("output_Cue2_PreR_Block_l2"=w144:i32)  [unwired: 11 in]
          n107 = call "BRig_dataLC_Cue2_PreR_Prob_l2.vi"() -> ("output_Cue2_PreR_Prob_l2"=w143:i32)  [unwired: 11 in]
          n108 = call "BRig_dataLC_Cue2_PreR_Delay_l2.vi"() -> ("output_Cue2_PreR_Delay_l2"=w142:i32)  [unwired: 11 in]
          n109 = call "BRig_dataLC_Cue2_PreR_DelayOpt_l2.vi"() -> ("output_Cue2_PreR_DelayOpt_l2"=w141:i32)  [unwired: 11 in]
          n110 = call "BRig_dataLC_Cue2_PreR_Count_l2.vi"() -> ("output_Cue2_PreR_Count_l2"=w140:i32)  [unwired: 11 in]
          n111 = Boolean To (0,1)(Boolean="LC_Cue_First_OnOff") -> (0, 1=w232:i16)
          n112 = Boolean To (0,1)(Boolean="LC_Cue_First_delayOpt") -> (0, 1=w231:i16)
          n113 = Boolean To (0,1)(Boolean="LC_Cue_PreR_OnOff") -> (0, 1=w230:i16)
          n114 = Boolean To (0,1)(Boolean="LC_Cue_PreR_delayOpt") -> (0, 1=w229:i16)
          n115 = Boolean To (0,1)(Boolean="LC_Cue_PostR_OnOff") -> (0, 1=w228:i16)
          n116 = Boolean To (0,1)(Boolean="LC_Cue_PostR_delayOpt") -> (0, 1=w227:i16)
          n117 = Boolean To (0,1)(Boolean="LC_Cue2_First_OnOff") -> (0, 1=w205:i16)
          n118 = Boolean To (0,1)(Boolean="LC_Cue2_First_delayOpt") -> (0, 1=w204:i16)
          n119 = Boolean To (0,1)(Boolean="LC_Cue2_PreR_OnOff") -> (0, 1=w203:i16)
          n120 = Boolean To (0,1)(Boolean="LC_Cue2_PreR_delayOpt") -> (0, 1=w202:i16)
          n121 = Boolean To (0,1)(Boolean="LC_Cue2_PostR_OnOff") -> (0, 1=w201:i16)
          n122 = Boolean To (0,1)(Boolean="LC_Cue2_PostR_delayOpt") -> (0, 1=w200:i16)
          n123 = To Unsigned Word Integer(number=w232) -> (unsigned 16bit integer=w226:u16)
          n124 = To Unsigned Word Integer(number=w231) -> (unsigned 16bit integer=w222:u16)
          n125 = To Unsigned Word Integer(number=w230) -> (unsigned 16bit integer=w220:u16)
          n126 = To Unsigned Word Integer(number=w229) -> (unsigned 16bit integer=w216:u16)
          n127 = To Unsigned Word Integer(number=w228) -> (unsigned 16bit integer=w214:u16)
          n128 = To Unsigned Word Integer(number=w227) -> (unsigned 16bit integer=w210:u16)
          n129 = To Unsigned Word Integer(number=w205) -> (unsigned 16bit integer=w193:u16)
          n130 = To Unsigned Word Integer(number=w204) -> (unsigned 16bit integer=w189:u16)
          n131 = To Unsigned Word Integer(number=w203) -> (unsigned 16bit integer=w187:u16)
          n132 = To Unsigned Word Integer(number=w202) -> (unsigned 16bit integer=w183:u16)
          n133 = To Unsigned Word Integer(number=w201) -> (unsigned 16bit integer=w181:u16)
          n134 = To Unsigned Word Integer(number=w200) -> (unsigned 16bit integer=w177:u16)
          n135 = call "BRig_dataLC_Cue_PostR_nRew1_l2.vi"() -> ("output_Cue_PostR_nRew1_l2"=w139:i32)  [unwired: 11 in]
          n136 = call "BRig_dataLC_Cue_PostR_nRew2_l2.vi"() -> ("output_Cue_PostR_nRew2_l2"=w138:i32)  [unwired: 11 in]
          n137 = call "BRig_dataLC_Cue2_PostR_nRew1_l2.vi"() -> ("output_Cue2_PostR_nRew1_l2"=w137:i32)  [unwired: 11 in]
          n138 = call "BRig_dataLC_Cue2_PostR_nRew2_l2.vi"() -> ("output_Cue2_PostR_nRew2_l2"=w136:i32)  [unwired: 11 in]
          n139 = Replace Array Subset(array=w240, new element #1=w207, index #1=w208, new element #2=w226, index #2=w158, new element #3="LC_Cue_First_Block", index #3=w159, new element #4="LC_Cue_First_Probability", index #4=w160, new element #5="LC_Cue_First_Tdelay", index #5=w161, new element #6=w222, index #6=w162, new element #7="LC_Cue_First_Count", index #7=w163, new element #8=w220, index #8=w164, new element #9="LC_Cue_PreR_Block", index #9=w165, new element #10="LC_Cue_PreR_Probability", index #10=w166, new element #11="LC_Cue_PreR_Tdelay", index #11=w167, new element #12=w216, index #12=w168, new element #13="LC_Cue_PreR_Count", index #13=w169, new element #14=w214, index #14=w170, new element #15="LC_Cue_PostR_Block", index #15=w171, new element #16="LC_Cue_PostR_Probability", index #16=w172, new element #17="LC_Cue_PostR_Tdelay", index #17=w173, new element #18=w210, index #18=w174, new element #19="LC_Cue_PostR_Count", index #19=w175, new element #20=w193, index #20=w157, new element #21="LC_Cue2_First_Block", index #21=w156, new element #22="LC_Cue2_First_Probability", index #22=w155, new element #23="LC_Cue2_First_Tdelay", index #23=w154, new element #24=w189, index #24=w153, new element #25="LC_Cue2_First_Count", index #25=w152, new element #26=w187, index #26=w151, new element #27="LC_Cue2_PreR_Block", index #27=w150, new element #28="LC_Cue2_PreR_Probability", index #28=w149, new element #29="LC_Cue2_PreR_Tdelay", index #29=w148, new element #30=w183, index #30=w147, new element #31="LC_Cue2_PreR_Count", index #31=w146, new element #32=w181, index #32=w145, new element #33="LC_Cue2_PostR_Block", index #33=w144, new element #34="LC_Cue2_PostR_Probability", index #34=w143, new element #35="LC_Cue2_PostR_Tdelay", index #35=w142, new element #36=w177, index #36=w141, new element #37="LC_Cue2_PostR_Count", index #37=w140, new element #38="LC_Cue_nRew1", index #38=w139, new element #39="LC_Cue_nRew2", index #39=w138, new element #40="LC_Cue2_nRew1", index #40=w137, new element #41="LC_Cue2_nRew2", index #41=w136) -> (w239:u16[])
        }
        frame 3 {
          n140 = call "BRig_dataLC_Selection_First_OnOff_l2.vi"() -> ("output_Selection_First_OnOff_l2"=w245:i32)  [unwired: 11 in]
          n141 = call "BRig_dataLC_Selection_First_Block_l2.vi"() -> ("output_Selection_First_Block_l2"=w246:i32)  [unwired: 11 in]
          n142 = call "BRig_dataLC_Selection_First_Prob_l2.vi"() -> ("output_Selection_First_Prob_l2"=w247:i32)  [unwired: 11 in]
          n143 = call "BRig_dataLC_Selection_First_Delay_l2.vi"() -> ("output_Selection_First_Delay_l2"=w248:i32)  [unwired: 11 in]
          n144 = call "BRig_dataLC_Selection_First_Count_l2.vi"() -> ("output_Selection_First_Count_l2"=w249:i32)  [unwired: 11 in]
          n145 = call "BRig_dataLC_Selection_PreR_OnOff_l2.vi"() -> ("output_Selection_PreR_OnOff_l2"=w250:i32)  [unwired: 11 in]
          n146 = call "BRig_dataLC_Selection_PreR_Block_l2.vi"() -> ("output_Selection_PreR_Block_l2"=w251:i32)  [unwired: 11 in]
          n147 = call "BRig_dataLC_Selection_PreR_Prob_l2.vi"() -> ("output_Selection_PreR_Prob_l2"=w252:i32)  [unwired: 11 in]
          n148 = call "BRig_dataLC_Selection_PreR_Delay_l2.vi"() -> ("output_Selection_PreR_Delay_l2"=w253:i32)  [unwired: 11 in]
          n149 = call "BRig_dataLC_Selection_PreR_Count_l2.vi"() -> ("output_Selection_PreR_Count_l2"=w254:i32)  [unwired: 11 in]
          n150 = call "BRig_dataLC_Selection_PostR_OnOff_l2.vi"() -> ("output_Selection_PostR_OnOff_l2"=w255:i32)  [unwired: 11 in]
          n151 = call "BRig_dataLC_Selection_PostR_Block_l2.vi"() -> ("output_Selection_PostR_Block_l2"=w256:i32)  [unwired: 11 in]
          n152 = call "BRig_dataLC_Selection_PostR_Prob_l2.vi"() -> ("output_Selection_PostR_Prob_l2"=w257:i32)  [unwired: 11 in]
          n153 = call "BRig_dataLC_Selection_PostR_Delay_l2.vi"() -> ("output_Selection_PostR_Delay_l2"=w258:i32)  [unwired: 11 in]
          n154 = call "BRig_dataLC_Selection_PostR_Count_l2.vi"() -> ("output_Selection_PostR_Count_l2"=w259:i32)  [unwired: 11 in]
          n155 = Boolean To (0,1)(Boolean="LC_Sel_First_OnOff") -> (0, 1=w280:i16)
          n156 = Boolean To (0,1)(Boolean="LC_Sel_PreR_OnOff") -> (0, 1=w279:i16)
          n157 = Boolean To (0,1)(Boolean="LC_Sel_PostR_OnOff") -> (0, 1=w278:i16)
          n158 = To Unsigned Word Integer(number=w280) -> (unsigned 16bit integer=w277:u16)
          n159 = To Unsigned Word Integer(number=w279) -> (unsigned 16bit integer=w272:u16)
          n160 = To Unsigned Word Integer(number=w278) -> (unsigned 16bit integer=w267:u16)
          n161 = call "BRig_dataLC_Selection_PostR_nRew1_l2.vi"() -> ("output_Selection_PostR_nRew1_l2"=w244:i32)  [unwired: 11 in]
          n162 = call "BRig_dataLC_Selection_PostR_nRew2_l2.vi"() -> ("output_Selection_PostR_nRew2_l2"=w243:i32)  [unwired: 11 in]
          n163 = Replace Array Subset(array=w285, new element #1=w261, index #1=w262, new element #2=w277, index #2=w245, new element #3="LC_Sel_First_Block", index #3=w246, new element #4="LC_Sel_First_Probability", index #4=w247, new element #5="LC_Sel_First_Tdelay", index #5=w248, new element #6="LC_Sel_First_Count", index #6=w249, new element #7=w272, index #7=w250, new element #8="LC_Sel_PreR_Block", index #8=w251, new element #9="LC_Sel_PreR_Probability", index #9=w252, new element #10="LC_Sel_PreR_Tdelay", index #10=w253, new element #11="LC_Sel_PreR_Count", index #11=w254, new element #12=w267, index #12=w255, new element #13="LC_Sel_PostR_Block", index #13=w256, new element #14="LC_Sel_PostR_Probability", index #14=w257, new element #15="LC_Sel_PostR_Tdelay", index #15=w258, new element #16="LC_Sel_PostR_Count", index #16=w259, new element #17="LC_Sel_nRew1", index #17=w244, new element #18="LC_Sel_nRew2", index #18=w243) -> (w284:u16[])
        }
        frame 4 {
          n164 = call "BRig_dataLC_Reward_OnOff_l2.vi"() -> ("output_Reward_OnOff_l2"=w286:i32)  [unwired: 11 in]
          n165 = call "BRig_dataLC_Reward_Block_l2.vi"() -> ("output_Reward_Block_l2"=w287:i32)  [unwired: 11 in]
          n166 = call "BRig_dataLC_Reward_Trial_l2.vi"() -> ("output_Reward_Trial_l2"=w288:i32)  [unwired: 11 in]
          n167 = call "BRig_dataLC_Reward_Prob_l2.vi"() -> ("output_Reward_Prob_l2"=w289:i32)  [unwired: 11 in]
          n168 = call "BRig_dataLC_Reward_Delay_l2.vi"() -> ("output_Reward_Delay_l2"=w290:i32)  [unwired: 11 in]
          n169 = call "BRig_dataLC_Wrong_OnOff_l2.vi"() -> ("output_Wrong_OnOff_l2"=w291:i32)  [unwired: 11 in]
          n170 = call "BRig_dataLC_Wrong_Block_l2.vi"() -> ("output_Wrong_Block_l2"=w292:i32)  [unwired: 11 in]
          n171 = call "BRig_dataLC_Wrong_Trial_l2.vi"() -> ("output_Wrong_Trial_l2"=w293:i32)  [unwired: 11 in]
          n172 = call "BRig_dataLC_Wrong_Prob_l2.vi"() -> ("output_Wrong_Prob_l2"=w294:i32)  [unwired: 11 in]
          n173 = call "BRig_dataLC_Wrong_Delay_l2.vi"() -> ("output_Wrong_Delay_l2"=w295:i32)  [unwired: 11 in]
          n174 = Boolean To (0,1)(Boolean="LC_Reward_OnOff") -> (0, 1=w310:i16)
          n175 = Boolean To (0,1)(Boolean="LC_Wrong_OnOff") -> (0, 1=w309:i16)
          n176 = To Unsigned Word Integer(number=w310) -> (unsigned 16bit integer=w308:u16)
          n177 = To Unsigned Word Integer(number=w309) -> (unsigned 16bit integer=w303:u16)
          n178 = Replace Array Subset(array=w314, new element #1=w297, index #1=w298, new element #2=w308, index #2=w286, new element #3="LC_Reward_Block", index #3=w287, new element #4="LC_Reward_Trial", index #4=w288, new element #5="LC_Reward_Probability", index #5=w289, new element #6="LC_Reward_Tdelay", index #6=w290, new element #7=w303, index #7=w291, new element #8="LC_Wrong_Block", index #8=w292, new element #9="LC_Wrong_Trial", index #9=w293, new element #10="LC_Wrong_Probability", index #10=w294, new element #11="LC_Wrong_Tdelay", index #11=w295) -> (w313:u16[])
        }
        frame 5 {
          w338 = 100.0 ("y")
          n179 = call "BRig_dataExp_LED_baseline_l2.vi"() -> ("output_LED_baseline_l2"=w315:i32)  [unwired: 11 in]
          n180 = call "BRig_dataExp_L_freq_l2.vi"() -> ("output_L_freq_l2"=w316:i32)  [unwired: 11 in]
          n181 = call "BRig_dataExp_L_T_l2.vi"() -> ("output_L_T_l2"=w317:i32)  [unwired: 11 in]
          n182 = call "BRig_dataExp_L_Tpeak_l2.vi"() -> ("output_L_Tpeak_l2"=w318:i32)  [unwired: 11 in]
          n183 = call "BRig_dataExp_L_Tshutter_l2.vi"() -> ("output_L_Tshutter_l2"=w319:i32)  [unwired: 11 in]
          n184 = call "BRig_dataExp_L_power_min_l2.vi"() -> ("output_L_power_min_l2"=w320:i32)  [unwired: 11 in]
          n185 = call "BRig_dataExp_L_power_max_l2.vi"() -> ("output_L_power_max_l2"=w321:i32)  [unwired: 11 in]
          n186 = call "BRig_dataExp_L_power_step_l2.vi"() -> ("output_L_power_step_l2"=w322:i32)  [unwired: 11 in]
          n187 = call "BRig_dataExp_L_Ttotal_l2.vi"() -> ("output_L_Ttotal_l2"=w323:i32)  [unwired: 11 in]
          n188 = Boolean To (0,1)(Boolean="LED_baseline") -> (0, 1=w350:i16)
          n189 = To Unsigned Word Integer(number=w350) -> (unsigned 16bit integer=w348:u16)
          n190 = Multiply(x="Laser_power_min", y=w338) -> (x*y=w342:dbl)
          n191 = Multiply(x="Laser_power_max", y=w338) -> (x*y=w344:dbl)
          n192 = Multiply(x="Laser_power_step", y=w338) -> (x*y=w347:dbl)
          n193 = Round To Nearest(number=w342) -> (nearest integer value=w341:dbl)
          n194 = Round To Nearest(number=w344) -> (nearest integer value=w343:dbl)
          n195 = Round To Nearest(number=w347) -> (nearest integer value=w346:dbl)
          n196 = To Unsigned Word Integer(number=w341) -> (unsigned 16bit integer=w335:u16)
          n197 = To Unsigned Word Integer(number=w343) -> (unsigned 16bit integer=w336:u16)
          n198 = To Unsigned Word Integer(number=w346) -> (unsigned 16bit integer=w337:u16)
          n199 = Add(x="Laser_T", y="Laser_Tshutter") -> (x+y=w330:u16)
          n200 = Replace Array Subset(array=w327, new element=w324, index=w325) -> (w326:u16[])
          n201 = Replace Array Subset(array=w329, new element #1=w348, index #1=w315, new element #2="Laser_Freq", index #2=w316, new element #3="Laser_T", index #3=w317, new element #4="Laser_Tpeak", index #4=w318, new element #5="Laser_Tshutter", index #5=w319, new element #6=w335, index #6=w320, new element #7=w336, index #7=w321, new element #8=w337, index #8=w322, new element #9=w330, index #9=w323) -> (w328:u16[])
        }
        frame 6 {
          n202 = call "BRig_dataExp_L_freq_l2.vi"() -> ("output_L_freq_l2"=w351:i32)  [unwired: 11 in]
          n203 = call "BRig_dataExp_L_T_l2.vi"() -> ("output_L_T_l2"=w352:i32)  [unwired: 11 in]
          n204 = call "BRig_dataExp_L_Tpeak_l2.vi"() -> ("output_L_Tpeak_l2"=w353:i32)  [unwired: 11 in]
          n205 = call "BRig_dataExp_L_Tshutter_l2.vi"() -> ("output_L_Tshutter_l2"=w354:i32)  [unwired: 11 in]
          n206 = Replace Array Subset(array=w358, new element=w355, index=w356) -> (w357:u16[])
          n207 = call "BRig_RT__Case_Idle__calc_LaserPulse.vi"("input_dataExp_L_Tshutter"=w354, "input_dataExp_L_Tpeak"=w353, "input_dataExp_L_T"=w352, "input_dataExp_L_freq"=w351, "input_dataExp"=w360) -> ("output_cluster"=→"LaserPulseTrain":cluster{u16[], u16[]})  [unwired: 6 in]
        }
      }
    }
    frame True {
      w517 = 100.0 ("y")
      n208 = call "BRig_dataLC_ENL_First_OnOff_l2.vi"() -> ("output_ENL_First_OnOff_l2"=w449:i32)  [unwired: 11 in]
      n209 = call "BRig_dataLC_ENL_First_Block_l2.vi"() -> ("output_ENL_First_Block_l2"=w448:i32)  [unwired: 11 in]
      n210 = call "BRig_dataLC_ENL_First_Prob_l2.vi"() -> ("output_ENL_First_Prob_l2"=w450:i32)  [unwired: 11 in]
      n211 = call "BRig_dataLC_ENL_First_Delay_l2.vi"() -> ("output_ENL_First_Delay_l2"=w451:i32)  [unwired: 11 in]
      n212 = call "BRig_dataLC_ENL_First_DelayOpt_l2.vi"() -> ("output_ENL_First_DelayOpt_l2"=w452:i32)  [unwired: 11 in]
      n213 = call "BRig_dataLC_ENL_First_Count_l2.vi"() -> ("output_ENL_First_Count_l2"=w453:i32)  [unwired: 11 in]
      n214 = call "BRig_dataLC_ENL_PreR_OnOff_l2.vi"() -> ("output_ENL_PreR_OnOff_l2"=w454:i32)  [unwired: 11 in]
      n215 = call "BRig_dataLC_ENL_PreR_Block_l2.vi"() -> ("output_ENL_PreR_Block_l2"=w455:i32)  [unwired: 11 in]
      n216 = call "BRig_dataLC_ENL_PreR_Prob_l2.vi"() -> ("output_ENL_PreR_Prob_l2"=w456:i32)  [unwired: 11 in]
      n217 = call "BRig_dataLC_ENL_PreR_Delay_l2.vi"() -> ("output_ENL_PreR_Delay_l2"=w457:i32)  [unwired: 11 in]
      n218 = call "BRig_dataLC_ENL_PreR_DelayOpt_l2.vi"() -> ("output_ENL_PreR_DelayOpt_l2"=w458:i32)  [unwired: 11 in]
      n219 = call "BRig_dataLC_ENL_PreR_Count_l2.vi"() -> ("output_ENL_PreR_Count_l2"=w459:i32)  [unwired: 11 in]
      n220 = call "BRig_dataLC_ENL_PostR_OnOff_l2.vi"() -> ("output_ENL_PostR_OnOff_l2"=w460:i32)  [unwired: 11 in]
      n221 = call "BRig_dataLC_ENL_PostR_Block_l2.vi"() -> ("output_ENL_PostR_Block_l2"=w461:i32)  [unwired: 11 in]
      n222 = call "BRig_dataLC_ENL_PostR_Prob_l2.vi"() -> ("output_ENL_PostR_Prob_l2"=w462:i32)  [unwired: 11 in]
      n223 = call "BRig_dataLC_ENL_PostR_Delay_l2.vi"() -> ("output_ENL_PostR_Delay_l2"=w463:i32)  [unwired: 11 in]
      n224 = call "BRig_dataLC_ENL_PostR_DelayOpt_l2.vi"() -> ("output_ENL_PostR_DelayOpt_l2"=w464:i32)  [unwired: 11 in]
      n225 = call "BRig_dataLC_ENL_PostR_Count_l2.vi"() -> ("output_ENL_PostR_Count_l2"=w465:i32)  [unwired: 11 in]
      n226 = call "BRig_dataLC_ENL2_First_OnOff_l2.vi"() -> ("output_ENL2_First_OnOff_l2"=w384:i32)  [unwired: 11 in]
      n227 = call "BRig_dataLC_ENL2_First_Block_l2.vi"() -> ("output_ENL2_First_Block_l2"=w383:i32)  [unwired: 11 in]
      n228 = call "BRig_dataLC_ENL2_First_Prob_l2.vi"() -> ("output_ENL2_First_Prob_l2"=w382:i32)  [unwired: 11 in]
      n229 = call "BRig_dataLC_ENL2_First_Delay_l2.vi"() -> ("output_ENL2_First_Delay_l2"=w381:i32)  [unwired: 11 in]
      n230 = call "BRig_dataLC_ENL2_First_DelayOpt_l2.vi"() -> ("output_ENL2_First_DelayOpt_l2"=w380:i32)  [unwired: 11 in]
      n231 = call "BRig_dataLC_ENL2_First_Count_l2.vi"() -> ("output_ENL2_First_Count_l2"=w379:i32)  [unwired: 11 in]
      n232 = call "BRig_dataLC_ENL2_PreR_OnOff_l2.vi"() -> ("output_ENL2_PreR_OnOff_l2"=w390:i32)  [unwired: 11 in]
      n233 = call "BRig_dataLC_ENL2_PreR_Block_l2.vi"() -> ("output_ENL2_PreR_Block_l2"=w389:i32)  [unwired: 11 in]
      n234 = call "BRig_dataLC_ENL2_PreR_Prob_l2.vi"() -> ("output_ENL2_PreR_Prob_l2"=w388:i32)  [unwired: 11 in]
      n235 = call "BRig_dataLC_ENL2_PreR_Delay_l2.vi"() -> ("output_ENL2_PreR_Delay_l2"=w387:i32)  [unwired: 11 in]
      n236 = call "BRig_dataLC_ENL2_PreR_DelayOpt_l2.vi"() -> ("output_ENL2_PreR_DelayOpt_l2"=w386:i32)  [unwired: 11 in]
      n237 = call "BRig_dataLC_ENL2_PreR_Count_l2.vi"() -> ("output_ENL2_PreR_Count_l2"=w385:i32)  [unwired: 11 in]
      n238 = call "BRig_dataLC_ENL2_PostR_OnOff_l2.vi"() -> ("output_ENL2_PostR_OnOff_l2"=w396:i32)  [unwired: 11 in]
      n239 = call "BRig_dataLC_ENL2_PostR_Block_l2.vi"() -> ("output_ENL2_PostR_Block_l2"=w395:i32)  [unwired: 11 in]
      n240 = call "BRig_dataLC_ENL2_PostR_Prob_l2.vi"() -> ("output_ENL2_PostR_Prob_l2"=w394:i32)  [unwired: 11 in]
      n241 = call "BRig_dataLC_ENL2_PostR_Delay_l2.vi"() -> ("output_ENL2_PostR_Delay_l2"=w393:i32)  [unwired: 11 in]
      n242 = call "BRig_dataLC_ENL2_PostR_DelayOpt_l2.vi"() -> ("output_ENL2_PostR_DelayOpt_l2"=w392:i32)  [unwired: 11 in]
      n243 = call "BRig_dataLC_ENL2_PostR_Count_l2.vi"() -> ("output_ENL2_PostR_Count_l2"=w391:i32)  [unwired: 11 in]
      n244 = Index Array(array=w531, index #1=w449, index #2=w448, index #3=w450, index #4=w451, index #5=w452, index #6=w453, index #7=w454, index #8=w455, index #9=w456, index #10=w457, index #11=w458, index #12=w459, index #13=w460, index #14=w461, index #15=w462, index #16=w463, index #17=w464, index #18=w465) -> (element #1=w603:u16, element #2=w602:u16, element #3=w601:u16, element #4=w600:u16, element #5=w599:u16, element #6=w598:u16, element #7=w597:u16, element #8=w596:u16, element #9=w595:u16, element #10=w594:u16, element #11=w593:u16, element #12=w592:u16, element #13=w591:u16, element #14=w590:u16, element #15=w589:u16, element #16=w588:u16, element #17=w587:u16, element #18=w586:u16)
      n245 = Index Array(array=w484, index #1=w384, index #2=w383, index #3=w382, index #4=w381, index #5=w380, index #6=w379, index #7=w390, index #8=w389, index #9=w388, index #10=w387, index #11=w386, index #12=w385, index #13=w396, index #14=w395, index #15=w394, index #16=w393, index #17=w392, index #18=w391) -> (element #1=w491:u16, element #2=w492:u16, element #3=w493:u16, element #4=w494:u16, element #5=w495:u16, element #6=w496:u16, element #7=w497:u16, element #8=w498:u16, element #9=w499:u16, element #10=w500:u16, element #11=w501:u16, element #12=w502:u16, element #13=w504:u16, element #14=w505:u16, element #15=w506:u16, element #16=w507:u16, element #17=w508:u16, element #18=w509:u16)
      n246 = Not Equal To 0?(x=w603) -> (x != 0?=w609:bool)
      n247 = Not Equal To 0?(x=w599) -> (x != 0?=w608:bool)
      n248 = Not Equal To 0?(x=w597) -> (x != 0?=w607:bool)
      n249 = Not Equal To 0?(x=w593) -> (x != 0?=w606:bool)
      n250 = Not Equal To 0?(x=w591) -> (x != 0?=w605:bool)
      n251 = Not Equal To 0?(x=w587) -> (x != 0?=w604:bool)
      n252 = local write "LC_ENL_First_OnOff"(w609) -> ()
      n253 = local write "LC_ENL_First_Block"(w602) -> ()
      n254 = local write "LC_ENL_First_Probability"(w601) -> ()
      n255 = local write "LC_ENL_First_Tdelay"(w600) -> ()
      n256 = local write "LC_ENL_First_delayOpt"(w608) -> ()
      n257 = local write "LC_ENL_First_Count"(w598) -> ()
      n258 = local write "LC_ENL_PreR_OnOff"(w607) -> ()
      n259 = local write "LC_ENL_PreR_Block"(w596) -> ()
      n260 = local write "LC_ENL_PreR_Probability"(w595) -> ()
      n261 = local write "LC_ENL_PreR_Tdelay"(w594) -> ()
      n262 = local write "LC_ENL_PreR_delayOpt"(w606) -> ()
      n263 = local write "LC_ENL_PreR_Count"(w592) -> ()
      n264 = local write "LC_ENL_PostR_OnOff"(w605) -> ()
      n265 = local write "LC_ENL_PostR_Block"(w590) -> ()
      n266 = local write "LC_ENL_PostR_Probability"(w589) -> ()
      n267 = local write "LC_ENL_PostR_Tdelay"(w588) -> ()
      n268 = local write "LC_ENL_PostR_delayOpt"(w604) -> ()
      n269 = local write "LC_ENL_PostR_Count"(w586) -> ()
      n270 = Not Equal To 0?(x=w491) -> (x != 0?=w512:bool)
      n271 = Not Equal To 0?(x=w495) -> (x != 0?=w513:bool)
      n272 = Not Equal To 0?(x=w497) -> (x != 0?=w511:bool)
      n273 = Not Equal To 0?(x=w501) -> (x != 0?=w514:bool)
      n274 = Not Equal To 0?(x=w504) -> (x != 0?=w510:bool)
      n275 = Not Equal To 0?(x=w508) -> (x != 0?=w503:bool)
      n276 = local write "LC_ENL2_First_OnOff"(w512) -> ()
      n277 = local write "LC_ENL2_First_Block"(w492) -> ()
      n278 = local write "LC_ENL2_First_Probability"(w493) -> ()
      n279 = local write "LC_ENL2_First_Tdelay"(w494) -> ()
      n280 = local write "LC_ENL2_First_delayOpt"(w513) -> ()
      n281 = local write "LC_ENL2_First_Count"(w496) -> ()
      n282 = local write "LC_ENL2_PreR_OnOff"(w511) -> ()
      n283 = local write "LC_ENL2_PreR_Block"(w498) -> ()
      n284 = local write "LC_ENL2_PreR_Probability"(w499) -> ()
      n285 = local write "LC_ENL2_PreR_Tdelay"(w500) -> ()
      n286 = local write "LC_ENL2_PreR_delayOpt"(w514) -> ()
      n287 = local write "LC_ENL2_PreR_Count"(w502) -> ()
      n288 = local write "LC_ENL2_PostR_OnOff"(w510) -> ()
      n289 = local write "LC_ENL2_PostR_Block"(w505) -> ()
      n290 = local write "LC_ENL2_PostR_Probability"(w506) -> ()
      n291 = local write "LC_ENL2_PostR_Tdelay"(w507) -> ()
      n292 = local write "LC_ENL2_PostR_delayOpt"(w503) -> ()
      n293 = local write "LC_ENL2_PostR_Count"(w509) -> ()
      n294 = call "BRig_dataLC_Cue_First_OnOff_l2.vi"() -> ("output_Cue_First_OnOff_l2"=w432:i32)  [unwired: 11 in]
      n295 = call "BRig_dataLC_Cue_First_Block_l2.vi"() -> ("output_Cue_First_Block_l2"=w430:i32)  [unwired: 11 in]
      n296 = call "BRig_dataLC_Cue_First_Prob_l2.vi"() -> ("output_Cue_First_Prob_l2"=w431:i32)  [unwired: 11 in]
      n297 = call "BRig_dataLC_Cue_First_Delay_l2.vi"() -> ("output_Cue_First_Delay_l2"=w433:i32)  [unwired: 11 in]
      n298 = call "BRig_dataLC_Cue_First_DelayOpt_l2.vi"() -> ("output_Cue_First_DelayOpt_l2"=w434:i32)  [unwired: 11 in]
      n299 = call "BRig_dataLC_Cue_First_Count_l2.vi"() -> ("output_Cue_First_Count_l2"=w435:i32)  [unwired: 11 in]
      n300 = call "BRig_dataLC_Cue_PreR_OnOff_l2.vi"() -> ("output_Cue_PreR_OnOff_l2"=w436:i32)  [unwired: 11 in]
      n301 = call "BRig_dataLC_Cue_PreR_Block_l2.vi"() -> ("output_Cue_PreR_Block_l2"=w437:i32)  [unwired: 11 in]
      n302 = call "BRig_dataLC_Cue_PreR_Prob_l2.vi"() -> ("output_Cue_PreR_Prob_l2"=w438:i32)  [unwired: 11 in]
      n303 = call "BRig_dataLC_Cue_PreR_Delay_l2.vi"() -> ("output_Cue_PreR_Delay_l2"=w439:i32)  [unwired: 11 in]
      n304 = call "BRig_dataLC_Cue_PreR_DelayOpt_l2.vi"() -> ("output_Cue_PreR_DelayOpt_l2"=w440:i32)  [unwired: 11 in]
      n305 = call "BRig_dataLC_Cue_PreR_Count_l2.vi"() -> ("output_Cue_PreR_Count_l2"=w441:i32)  [unwired: 11 in]
      n306 = call "BRig_dataLC_Cue_PostR_OnOff_l2.vi"() -> ("output_Cue_PostR_OnOff_l2"=w442:i32)  [unwired: 11 in]
      n307 = call "BRig_dataLC_Cue_PostR_Block_l2.vi"() -> ("output_Cue_PostR_Block_l2"=w443:i32)  [unwired: 11 in]
      n308 = call "BRig_dataLC_Cue_PostR_Prob_l2.vi"() -> ("output_Cue_PostR_Prob_l2"=w444:i32)  [unwired: 11 in]
      n309 = call "BRig_dataLC_Cue_PostR_Delay_l2.vi"() -> ("output_Cue_PostR_Delay_l2"=w445:i32)  [unwired: 11 in]
      n310 = call "BRig_dataLC_Cue_PostR_DelayOpt_l2.vi"() -> ("output_Cue_PostR_DelayOpt_l2"=w446:i32)  [unwired: 11 in]
      n311 = call "BRig_dataLC_Cue_PostR_Count_l2.vi"() -> ("output_Cue_PostR_Count_l2"=w447:i32)  [unwired: 11 in]
      n312 = call "BRig_dataExp_LED_baseline_l2.vi"() -> ("output_LED_baseline_l2"=w404:i32)  [unwired: 11 in]
      n313 = call "BRig_dataExp_L_freq_l2.vi"() -> ("output_L_freq_l2"=w403:i32)  [unwired: 11 in]
      n314 = call "BRig_dataExp_L_T_l2.vi"() -> ("output_L_T_l2"=w402:i32)  [unwired: 11 in]
      n315 = call "BRig_dataExp_L_Tpeak_l2.vi"() -> ("output_L_Tpeak_l2"=w401:i32)  [unwired: 11 in]
      n316 = call "BRig_dataExp_L_Tshutter_l2.vi"() -> ("output_L_Tshutter_l2"=w400:i32)  [unwired: 11 in]
      n317 = call "BRig_dataExp_L_power_min_l2.vi"() -> ("output_L_power_min_l2"=w399:i32)  [unwired: 11 in]
      n318 = call "BRig_dataExp_L_power_max_l2.vi"() -> ("output_L_power_max_l2"=w398:i32)  [unwired: 11 in]
      n319 = call "BRig_dataExp_L_power_step_l2.vi"() -> ("output_L_power_step_l2"=w397:i32)  [unwired: 11 in]
      n320 = Index Array(array=w531, index #1=w432, index #2=w430, index #3=w431, index #4=w433, index #5=w434, index #6=w435, index #7=w436, index #8=w437, index #9=w438, index #10=w439, index #11=w440, index #12=w441, index #13=w442, index #14=w443, index #15=w444, index #16=w445, index #17=w446, index #18=w447) -> (element #1=w579:u16, element #2=w578:u16, element #3=w577:u16, element #4=w576:u16, element #5=w575:u16, element #6=w574:u16, element #7=w573:u16, element #8=w572:u16, element #9=w571:u16, element #10=w570:u16, element #11=w569:u16, element #12=w568:u16, element #13=w567:u16, element #14=w566:u16, element #15=w565:u16, element #16=w564:u16, element #17=w563:u16, element #18=w562:u16)
      n321 = Index Array(array=w484, index #1=w404, index #2=w403, index #3=w402, index #4=w401, index #5=w400, index #6=w399, index #7=w398, index #8=w397) -> (element #1=w530:u16, element #2=w528:u16, element #3=w527:u16, element #4=w526:u16, element #5=w525:u16, element #6=w524:u16, element #7=w523:u16, element #8=w522:u16)
      n322 = To Double Precision Float(number=w524) -> (double precision float=w521:dbl)
      n323 = To Double Precision Float(number=w523) -> (double precision float=w516:dbl)
      n324 = To Double Precision Float(number=w522) -> (double precision float=w515:dbl)
      n325 = Not Equal To 0?(x=w579) -> (x != 0?=w585:bool)
      n326 = Not Equal To 0?(x=w575) -> (x != 0?=w584:bool)
      n327 = Not Equal To 0?(x=w573) -> (x != 0?=w583:bool)
      n328 = Not Equal To 0?(x=w569) -> (x != 0?=w582:bool)
      n329 = Not Equal To 0?(x=w567) -> (x != 0?=w581:bool)
      n330 = Not Equal To 0?(x=w563) -> (x != 0?=w580:bool)
      n331 = Divide(x=w521, y=w517) -> (x/y=w520:dbl)
      n332 = Divide(x=w516, y=w517) -> (x/y=w519:dbl)
      n333 = Divide(x=w515, y=w517) -> (x/y=w518:dbl)
      n334 = local write "LC_Cue_First_OnOff"(w585) -> ()
      n335 = local write "LC_Cue_First_Block"(w578) -> ()
      n336 = local write "LC_Cue_First_Probability"(w577) -> ()
      n337 = local write "LC_Cue_First_Tdelay"(w576) -> ()
      n338 = local write "LC_Cue_First_delayOpt"(w584) -> ()
      n339 = local write "LC_Cue_First_Count"(w574) -> ()
      n340 = local write "LC_Cue_PreR_OnOff"(w583) -> ()
      n341 = local write "LC_Cue_PreR_Block"(w572) -> ()
      n342 = local write "LC_Cue_PreR_Probability"(w571) -> ()
      n343 = local write "LC_Cue_PreR_Tdelay"(w570) -> ()
      n344 = local write "LC_Cue_PreR_delayOpt"(w582) -> ()
      n345 = local write "LC_Cue_PreR_Count"(w568) -> ()
      n346 = local write "LC_Cue_PostR_OnOff"(w581) -> ()
      n347 = local write "LC_Cue_PostR_Block"(w566) -> ()
      n348 = local write "LC_Cue_PostR_Probability"(w565) -> ()
      n349 = local write "LC_Cue_PostR_Tdelay"(w564) -> ()
      n350 = local write "LC_Cue_PostR_delayOpt"(w580) -> ()
      n351 = local write "LC_Cue_PostR_Count"(w562) -> ()
      n352 = Not Equal To 0?(x=w530) -> (x != 0?=w529:bool)
      n353 = call "BRig_dataLC_Cue2_First_OnOff_l2.vi"() -> ("output_Cue2_First_OnOff_l2"=w378:i32)  [unwired: 11 in]
      n354 = call "BRig_dataLC_Cue2_First_Block_l2.vi"() -> ("output_Cue2_First_Block_l2"=w377:i32)  [unwired: 11 in]
      n355 = call "BRig_dataLC_Cue2_First_Prob_l2.vi"() -> ("output_Cue2_First_Prob_l2"=w376:i32)  [unwired: 11 in]
      n356 = call "BRig_dataLC_Cue2_First_Delay_l2.vi"() -> ("output_Cue2_First_Delay_l2"=w375:i32)  [unwired: 11 in]
      n357 = call "BRig_dataLC_Cue2_First_DelayOpt_l2.vi"() -> ("output_Cue2_First_DelayOpt_l2"=w374:i32)  [unwired: 11 in]
      n358 = call "BRig_dataLC_Cue2_First_Count_l2.vi"() -> ("output_Cue2_First_Count_l2"=w373:i32)  [unwired: 11 in]
      n359 = call "BRig_dataLC_Cue2_PostR_OnOff_l2.vi"() -> ("output_Cue2_PostR_OnOff_l2"=w372:i32)  [unwired: 11 in]
      n360 = call "BRig_dataLC_Cue2_PostR_Block_l2.vi"() -> ("output_Cue2_PostR_Block_l2"=w371:i32)  [unwired: 11 in]
      n361 = call "BRig_dataLC_Cue2_PostR_Prob_l2.vi"() -> ("output_Cue2_PostR_Prob_l2"=w370:i32)  [unwired: 11 in]
      n362 = call "BRig_dataLC_Cue2_PostR_Delay_l2.vi"() -> ("output_Cue2_PostR_Delay_l2"=w369:i32)  [unwired: 11 in]
      n363 = call "BRig_dataLC_Cue2_PostR_DelayOpt_l2.vi"() -> ("output_Cue2_PostR_DelayOpt_l2"=w368:i32)  [unwired: 11 in]
      n364 = call "BRig_dataLC_Cue2_PostR_Count_l2.vi"() -> ("output_Cue2_PostR_Count_l2"=w367:i32)  [unwired: 11 in]
      n365 = call "BRig_dataLC_Cue2_PreR_OnOff_l2.vi"() -> ("output_Cue2_PreR_OnOff_l2"=w366:i32)  [unwired: 11 in]
      n366 = call "BRig_dataLC_Cue2_PreR_Block_l2.vi"() -> ("output_Cue2_PreR_Block_l2"=w365:i32)  [unwired: 11 in]
      n367 = call "BRig_dataLC_Cue2_PreR_Prob_l2.vi"() -> ("output_Cue2_PreR_Prob_l2"=w364:i32)  [unwired: 11 in]
      n368 = call "BRig_dataLC_Cue2_PreR_Delay_l2.vi"() -> ("output_Cue2_PreR_Delay_l2"=w363:i32)  [unwired: 11 in]
      n369 = call "BRig_dataLC_Cue2_PreR_DelayOpt_l2.vi"() -> ("output_Cue2_PreR_DelayOpt_l2"=w362:i32)  [unwired: 11 in]
      n370 = call "BRig_dataLC_Cue2_PreR_Count_l2.vi"() -> ("output_Cue2_PreR_Count_l2"=w361:i32)  [unwired: 11 in]
      n371 = local write "LED_baseline"(w529) -> ()
      n372 = local write "Laser_Freq"(w528) -> ()
      n373 = local write "Laser_T"(w527) -> ()
      n374 = local write "Laser_Tpeak"(w526) -> ()
      n375 = local write "Laser_Tshutter"(w525) -> ()
      n376 = local write "Laser_power_min"(w520) -> ()
      n377 = local write "Laser_power_max"(w519) -> ()
      n378 = local write "Laser_power_step"(w518) -> ()
      n379 = Index Array(array=w484, index #1=w378, index #2=w377, index #3=w376, index #4=w375, index #5=w374, index #6=w373, index #7=w372, index #8=w371, index #9=w370, index #10=w369, index #11=w368, index #12=w367, index #13=w366, index #14=w365, index #15=w364, index #16=w363, index #17=w362, index #18=w361) -> (element #1=w485:u16, element #2=w480:u16, element #3=w479:u16, element #4=w478:u16, element #5=w486:u16, element #6=w481:u16, element #7=w487:u16, element #8=w475:u16, element #9=w474:u16, element #10=w473:u16, element #11=w488:u16, element #12=w472:u16, element #13=w489:u16, element #14=w469:u16, element #15=w468:u16, element #16=w467:u16, element #17=w490:u16, element #18=w466:u16)
      n380 = call "BRig_dataLC_Selection_First_OnOff_l2.vi"() -> ("output_Selection_First_OnOff_l2"=w429:i32)  [unwired: 11 in]
      n381 = call "BRig_dataLC_Selection_First_Block_l2.vi"() -> ("output_Selection_First_Block_l2"=w428:i32)  [unwired: 11 in]
      n382 = call "BRig_dataLC_Selection_First_Prob_l2.vi"() -> ("output_Selection_First_Prob_l2"=w427:i32)  [unwired: 11 in]
      n383 = call "BRig_dataLC_Selection_First_Delay_l2.vi"() -> ("output_Selection_First_Delay_l2"=w426:i32)  [unwired: 11 in]
      n384 = call "BRig_dataLC_Selection_First_Count_l2.vi"() -> ("output_Selection_First_Count_l2"=w425:i32)  [unwired: 11 in]
      n385 = call "BRig_dataLC_Selection_PreR_OnOff_l2.vi"() -> ("output_Selection_PreR_OnOff_l2"=w424:i32)  [unwired: 11 in]
      n386 = call "BRig_dataLC_Selection_PreR_Block_l2.vi"() -> ("output_Selection_PreR_Block_l2"=w423:i32)  [unwired: 11 in]
      n387 = call "BRig_dataLC_Selection_PreR_Prob_l2.vi"() -> ("output_Selection_PreR_Prob_l2"=w422:i32)  [unwired: 11 in]
      n388 = call "BRig_dataLC_Selection_PreR_Delay_l2.vi"() -> ("output_Selection_PreR_Delay_l2"=w421:i32)  [unwired: 11 in]
      n389 = call "BRig_dataLC_Selection_PreR_Count_l2.vi"() -> ("output_Selection_PreR_Count_l2"=w420:i32)  [unwired: 11 in]
      n390 = call "BRig_dataLC_Selection_PostR_OnOff_l2.vi"() -> ("output_Selection_PostR_OnOff_l2"=w419:i32)  [unwired: 11 in]
      n391 = call "BRig_dataLC_Selection_PostR_Block_l2.vi"() -> ("output_Selection_PostR_Block_l2"=w418:i32)  [unwired: 11 in]
      n392 = call "BRig_dataLC_Selection_PostR_Prob_l2.vi"() -> ("output_Selection_PostR_Prob_l2"=w417:i32)  [unwired: 11 in]
      n393 = call "BRig_dataLC_Selection_PostR_Delay_l2.vi"() -> ("output_Selection_PostR_Delay_l2"=w416:i32)  [unwired: 11 in]
      n394 = call "BRig_dataLC_Selection_PostR_Count_l2.vi"() -> ("output_Selection_PostR_Count_l2"=w415:i32)  [unwired: 11 in]
      n395 = call "BRig_dataLC_Reward_OnOff_l2.vi"() -> ("output_Reward_OnOff_l2"=w405:i32)  [unwired: 11 in]
      n396 = call "BRig_dataLC_Reward_Block_l2.vi"() -> ("output_Reward_Block_l2"=w406:i32)  [unwired: 11 in]
      n397 = call "BRig_dataLC_Reward_Trial_l2.vi"() -> ("output_Reward_Trial_l2"=w407:i32)  [unwired: 11 in]
      n398 = call "BRig_dataLC_Reward_Prob_l2.vi"() -> ("output_Reward_Prob_l2"=w408:i32)  [unwired: 11 in]
      n399 = call "BRig_dataLC_Reward_Delay_l2.vi"() -> ("output_Reward_Delay_l2"=w409:i32)  [unwired: 11 in]
      n400 = call "BRig_dataLC_Wrong_OnOff_l2.vi"() -> ("output_Wrong_OnOff_l2"=w410:i32)  [unwired: 11 in]
      n401 = call "BRig_dataLC_Wrong_Block_l2.vi"() -> ("output_Wrong_Block_l2"=w411:i32)  [unwired: 11 in]
      n402 = call "BRig_dataLC_Wrong_Trial_l2.vi"() -> ("output_Wrong_Trial_l2"=w412:i32)  [unwired: 11 in]
      n403 = call "BRig_dataLC_Wrong_Prob_l2.vi"() -> ("output_Wrong_Prob_l2"=w413:i32)  [unwired: 11 in]
      n404 = call "BRig_dataLC_Wrong_Delay_l2.vi"() -> ("output_Wrong_Delay_l2"=w414:i32)  [unwired: 11 in]
      n405 = Not Equal To 0?(x=w485) -> (x != 0?=w483:bool)
      n406 = Not Equal To 0?(x=w486) -> (x != 0?=w482:bool)
      n407 = Not Equal To 0?(x=w487) -> (x != 0?=w476:bool)
      n408 = Not Equal To 0?(x=w488) -> (x != 0?=w477:bool)
      n409 = Not Equal To 0?(x=w489) -> (x != 0?=w471:bool)
      n410 = Not Equal To 0?(x=w490) -> (x != 0?=w470:bool)
      n411 = Index Array(array=w531, index #1=w405, index #2=w406, index #3=w407, index #4=w408, index #5=w409, index #6=w410, index #7=w411, index #8=w412, index #9=w413, index #10=w414) -> (element #1=w541:u16, element #2=w540:u16, element #3=w539:u16, element #4=w538:u16, element #5=w537:u16, element #6=w536:u16, element #7=w535:u16, element #8=w534:u16, element #9=w533:u16, element #10=w532:u16)
      n412 = local write "LC_Cue2_First_OnOff"(w483) -> ()
      n413 = local write "LC_Cue2_First_Block"(w480) -> ()
      n414 = local write "LC_Cue2_First_Probability"(w479) -> ()
      n415 = local write "LC_Cue2_First_Tdelay"(w478) -> ()
      n416 = local write "LC_Cue2_First_delayOpt"(w482) -> ()
      n417 = local write "LC_Cue2_First_Count"(w481) -> ()
      n418 = local write "LC_Cue2_PreR_OnOff"(w476) -> ()
      n419 = local write "LC_Cue2_PreR_Block"(w475) -> ()
      n420 = local write "LC_Cue2_PreR_Probability"(w474) -> ()
      n421 = local write "LC_Cue2_PreR_Tdelay"(w473) -> ()
      n422 = local write "LC_Cue2_PreR_delayOpt"(w477) -> ()
      n423 = local write "LC_Cue2_PreR_Count"(w472) -> ()
      n424 = local write "LC_Cue2_PostR_OnOff"(w471) -> ()
      n425 = local write "LC_Cue2_PostR_Block"(w469) -> ()
      n426 = local write "LC_Cue2_PostR_Probability"(w468) -> ()
      n427 = local write "LC_Cue2_PostR_Tdelay"(w467) -> ()
      n428 = local write "LC_Cue2_PostR_delayOpt"(w470) -> ()
      n429 = local write "LC_Cue2_PostR_Count"(w466) -> ()
      n430 = Index Array(array=w531, index #1=w429, index #2=w428, index #3=w427, index #4=w426, index #5=w425, index #6=w424, index #7=w423, index #8=w422, index #9=w421, index #10=w420, index #11=w419, index #12=w418, index #13=w417, index #14=w416, index #15=w415) -> (element #1=w558:u16, element #2=w557:u16, element #3=w556:u16, element #4=w555:u16, element #5=w554:u16, element #6=w553:u16, element #7=w552:u16, element #8=w551:u16, element #9=w550:u16, element #10=w549:u16, element #11=w548:u16, element #12=w547:u16, element #13=w546:u16, element #14=w545:u16, element #15=w544:u16)
      n431 = Not Equal To 0?(x=w541) -> (x != 0?=w543:bool)
      n432 = Not Equal To 0?(x=w536) -> (x != 0?=w542:bool)
      n433 = Not Equal To 0?(x=w558) -> (x != 0?=w561:bool)
      n434 = Not Equal To 0?(x=w553) -> (x != 0?=w560:bool)
      n435 = Not Equal To 0?(x=w548) -> (x != 0?=w559:bool)
      n436 = local write "LC_Reward_OnOff"(w543) -> ()
      n437 = local write "LC_Reward_Block"(w540) -> ()
      n438 = local write "LC_Reward_Trial"(w539) -> ()
      n439 = local write "LC_Reward_Probability"(w538) -> ()
      n440 = local write "LC_Reward_Tdelay"(w537) -> ()
      n441 = local write "LC_Wrong_OnOff"(w542) -> ()
      n442 = local write "LC_Wrong_Block"(w535) -> ()
      n443 = local write "LC_Wrong_Trial"(w534) -> ()
      n444 = local write "LC_Wrong_Probability"(w533) -> ()
      n445 = local write "LC_Wrong_Tdelay"(w532) -> ()
      n446 = local write "LC_Sel_First_OnOff"(w561) -> ()
      n447 = local write "LC_Sel_First_Block"(w557) -> ()
      n448 = local write "LC_Sel_First_Probability"(w556) -> ()
      n449 = local write "LC_Sel_First_Tdelay"(w555) -> ()
      n450 = local write "LC_Sel_First_Count"(w554) -> ()
      n451 = local write "LC_Sel_PreR_OnOff"(w560) -> ()
      n452 = local write "LC_Sel_PreR_Block"(w552) -> ()
      n453 = local write "LC_Sel_PreR_Probability"(w551) -> ()
      n454 = local write "LC_Sel_PreR_Tdelay"(w550) -> ()
      n455 = local write "LC_Sel_PreR_Count"(w549) -> ()
      n456 = local write "LC_Sel_PostR_OnOff"(w559) -> ()
      n457 = local write "LC_Sel_PostR_Block"(w547) -> ()
      n458 = local write "LC_Sel_PostR_Probability"(w546) -> ()
      n459 = local write "LC_Sel_PostR_Tdelay"(w545) -> ()
      n460 = local write "LC_Sel_PostR_Count"(w544) -> ()
    }
  }
  "output_dataLC" <- w4
  "output_dataExp" <- w1
